vi "Working Lock-In.vi"() -> ()   [LabVIEW 2013, in "Lock-In Variable Channels_2.lvclass"]
uses:
  Lock-In Variable Channels_2.lvclass
  XControl_next Folder/XControl_next.xctl
  Joe's Lock-In Files/Lockin-4461_3.0 4461-4462 Multichannel Folder/DAQ-Lockin-SubVI/Lock-in Globles Multiple Inputs and Outputs.vi
  Joe's Lock-In Files/Global Value_charles.vi
panel:
  out "first_run?":dbl
  out "Phase&Tc Control 2":T1(array[cluster])=[{"Phase"=0.0, "Time constant"=0.1, "Set Tc"=FALSE, "Autophase"=FALSE, "Order"=2.0}, {"Phase"=0.0, "Time constant"=0.1, "Set Tc"=FALSE, "Autophase"=FALSE, "Order"=2.0}, {"Phase"=0.0, "Time constant"=0.1, "Set Tc"=FALSE, "Autophase"=FALSE, "Order"=2.0}, {"Phase"=0.0, "Time constant"=0.1, "Set Tc"=FALSE, "Autophase"=FALSE, "Order"=2.0}, {"Phase"=0.0, "Time constant"=0.1, "Set Tc"=FALSE, "Autophase"=FALSE, "Order"=2.0}, {"Phase"=0.0, "Time constant"=0.1, "Set Tc"=FALSE, "Autophase"=FALSE, "Order"=2.0}, {"Phase"=0.0, "Time constant"=0.1, "Set Tc"=FALSE, "Autophase"=FALSE, "Order"=2.0}, {"Phase"=0.0, "Time constant"=0.1, "Set Tc"=FALSE, "Autophase"=FALSE, "Order"=2.0}, {"Phase"=0.0, "Time constant"=0.1, "Set Tc"=FALSE, "Autophase"=FALSE, "Order"=2.0}, {"Phase"=0.0, "Time constant"=0.1, "Set Tc"=FALSE, "Autophase"=FALSE, "Order"=2.0}, {"Phase"=0.0, "Time constant"=0.1, "Set Tc"=FALSE, "Autophase"=FALSE, "Order"=2.0}, {"Phase"=0.0, "Time constant"=0.1, "Set Tc"=FALSE, "Autophase"=FALSE, "Order"=2.0}, {"Phase"=0.0, "Time constant"=0.1, "Set Tc"=FALSE, "Autophase"=FALSE, "Order"=2.0}, {"Phase"=0.0, "Time constant"=0.1, "Set Tc"=FALSE, "Autophase"=FALSE, "Order"=2.0}, {"Phase"=0.0, "Time constant"=0.1, "Set Tc"=FALSE, "Autophase"=FALSE, "Order"=2.0}, {"Phase"=0.0, "Time constant"=0.1, "Set Tc"=FALSE, "Autophase"=FALSE, "Order"=2.0}, {"Phase"=0.0, "Time constant"=0.1, "Set Tc"=FALSE, "Autophase"=FALSE, "Order"=2.0}] {"Phase" min=0.0 max=360.0 scale=0.0..360.0}
  in  "Boolean_event":bool
  out "Multiple Indicator":bool
  out "Phase indicator":bool
  out "Signal indicator":bool
  out "loop counter":dbl
  out "Amp. button 2":bool
  out "DC button 2":bool
  out "OK Button 2":bool
  out "Boolean_panel3":bool
  out "Boolean_panel2":bool
  out "Numeric_Channel":dbl
  in  "XControl_next":dbl(xcontrol)
  in  "Display":u16(ring) items=["X and Y", "R and Theta"]
  in  "stop":bool
  out "Display 2":string="-000.000000       V"
  out "Display 1":string="-000.000000       V"
  out "Results":dbl[][](array[numeric])=[[1.1085752698169061e-06, 8.970523484593692e-07, 1.426058219262487e-06, 38.9795731407906], [0.009851325382064164, -0.0009794262328395094, 0.009899893308964286, -5.677731707079707], [1.3085970697368273e-06, 7.35860824175527e-07, 1.5013052466038e-06, 29.35026849878307], [2.653910755996262e-06, 1.0145343098285082e-06, 2.8412184299366806e-06, 20.9208047375633], [-6.086289413703597e-07, 1.180787094252328e-06, 1.3284153530528245e-06, 117.2685442231227], [2.777937660299593e-06, 8.877049230863689e-07, 2.9163260577278655e-06, 17.721560078700946]]
  in  "Remote":bool
  out "Backlog":u8(slide) scale=0.0..100.0
  out "Signal":dbl[][](array[numeric])
  in  "Tab Control":T2(tab)=enum."Input Signals"
  in  "Lockin Display A":i16(slide)=1 scale=1.0..18.0
  out "Display X (or R) A":dbl[](graph)=[6.670498573825442e-08, 5.368688471545208e-07, -5.088691339548878e-07, -2.5730186693772355e-06, -1.7991552027288684e-06, -1.923632216975614e-06, -1.4467888340965616e-06, -8.796097429790696e-07, -1.269884182091489e-06, -2.961296758715229e-06, -1.9896471500029525e-06, -2.992785692825242e-06, -1.7650822258067036e-06, -2.6746621457151217e-06, -1.8077634796781362e-07, -2.8403618391177364e-06, 1.7191093719052563e-06, -4.095627199796772e-06, 1.0350053729206764e-07, -3.2952403320842463e-06, 4.027147024255837e-07, -3.217883708836871e-06, -3.1404111038198314e-07, -2.722157981623261e-06, -2.3343431458291097e-06, -1.6493479166701816e-06, -1.1867860941043085e-06, -1.6312467794017544e-06, -1.924154413394931e-06, -1.9805292725153245e-06, 7.32780599223683e-07, -1.9269225043914707e-06, -1.9357725457213794e-06, -2.2334144149538824e-06, -4.935649750003306e-09, -8.436124644364356e-07, -3.307435264761252e-07, -2.3962904127030663e-06, -5.02686543328057e-07, -2.0819204665377523e-07, -6.016691845226929e-07, -3.3346199078653027e-06, -2.3438333439908954e-06, -2.6393322677123663e-06, 4.3707871692753315e-07, -1.955570749471345e-06, -1.0959726290001432e-06, -3.3918492580454637e-06, 2.46039910232935e-07, -1.9940219874551605e-06, -3.6795795043347265e-07, -2.45582698051919e-06, 4.455716118537976e-08, -1.5262074036175926e-06, 2.820130220284548e-07, -1.0569110213571934e-06, -2.3607453703924565e-07, -3.055913228346468e-06, -1.650377972048181e-06, -1.8932005087329695e-06, 5.914078647979998e-07, -1.3508504110029581e-06, -1.7773157019895033e-06, -1.433545330477821e-06, 5.165591171148216e-07, -2.6433445727486453e-07, -5.167671626878888e-07, -6.055573834856804e-07, -3.980981522485872e-07, -9.728044362515663e-07, -1.1758902512983826e-07, -1.6542257074006194e-06, -1.0669038863728946e-06, -1.1680190342438217e-06, -1.4347012124266572e-06, -2.233685467775109e-06, -9.173892627620104e-07, -1.3057567635081897e-06, -5.961972413873471e-07, -1.0467491581646199e-06, -1.5607311611567676e-06, -2.1330252927991802e-06, -1.2651497555792722e-06, -1.5740108560218413e-06, -8.450526108735602e-07, -1.1403712648585578e-07, -1.3527516308023321e-06, -8.078702051960308e-07, -9.409207938670527e-07, -1.5548207904995552e-06, -1.1518398452053984e-06, -1.3918660560555396e-06, -2.0931739723389586e-06, -2.2147164239668027e-06, -3.366260220930173e-06, -1.031323116424528e-06, -6.179742691405814e-07, -2.9460438011649747e-06, -1.1400531118409205e-06, -1.484088446722104e-07, -2.6518751029251362e-06, -4.097924835402338e-07, -2.057919982499709e-06, -2.715956482323881e-07, -6.940554229154257e-07, -7.522735265241387e-07, -7.335964599058371e-07, -2.8600098545973234e-07, -3.4843824827197703e-06, -1.44911890347727e-06, -1.225529253887876e-06, -6.736912990276699e-07, -1.6691842479645122e-06, -2.1938552441526384e-06, -1.4997095470240344e-06, -1.0375533719089362e-06, -1.1301499898056886e-06, -1.4793551793585697e-06, -2.5259160810447276e-06, 3.491557595541023e-07, -1.0993167478065809e-06, -1.068633016308054e-06, -8.806665544284457e-07, 9.238520373506171e-08, -7.19060141525052e-07, -1.22036415098872e-07, -9.144936655123115e-07, -9.321502892559434e-07, -1.8082361748005226e-06, -8.045321826052708e-07, -4.6816599025933015e-07, -1.201527764455396e-06, -9.433090453378502e-07, 5.799679027359041e-07, -2.6489856161776193e-06, 3.022449142514117e-07, 1.1085752698169061e-06, 0.0, 0.0, 0.0, 0.0, 0.0, 0.0, 0.0, 0.0, 0.0, 0.0, 0.0, 0.0, 0.0, 0.0, 0.0, 0.0, 0.0, 0.0, 0.0, 0.0, 0.0, 0.0, 0.0, 0.0, 0.0, 0.0, 0.0, 0.0, 0.0, 0.0, 0.0, 0.0, 0.0, 0.0, 0.0, 0.0, 0.0, 0.0, 0.0, 0.0, 0.0, 0.0, 0.0, 0.0, 0.0, 0.0, 0.0, 0.0, 0.0, 0.0, 0.0, 0.0, 0.0, 0.0, 0.0, 0.0, 0.0, 0.0, 0.0, 0.0, 0.0, 0.0, 0.0]
  out "Display Y (or Theta) A":dbl[](graph)=[1.0286335437287416e-07, 7.146914430049907e-07, 9.19371053154206e-07, -2.7527637468034014e-07, 9.764685600495431e-07, 2.16329849650388e-06, 6.18754045208451e-07, 1.0259603006949609e-06, 2.579095660939101e-07, 1.498736189536387e-06, 1.7791032720161242e-06, 8.722478978782919e-07, 1.179386006030635e-06, 1.3778637608132363e-06, -2.0572071085454253e-07, 7.203248036070591e-07, 6.266561030444089e-07, 1.2536548086139658e-06, -1.6258653973034804e-07, 1.9278115524532664e-06, 5.186481319325723e-07, 8.153605722202512e-07, 5.135548811901674e-07, 1.4550446823081113e-06, 3.3380469223525346e-07, 1.230454826405213e-06, 1.0885651868509204e-06, 1.5786789143860278e-06, 9.455455089747191e-07, 1.2571272379312255e-06, 2.1014333516181865e-06, 6.607774722121163e-07, 4.822838575243949e-07, 9.038988408693548e-07, 1.33469270633984e-06, 6.455872176713377e-07, 5.666811221789705e-07, 1.0640103180436064e-06, 1.4303236294814581e-06, 6.967580372586826e-07, 6.136341751512432e-07, 7.422882569256587e-07, 5.883881949852455e-07, 1.997573203066393e-06, 5.108273813688291e-07, 1.7950225152410556e-06, 1.221042319602369e-06, 9.86349423686866e-07, 9.54101478401993e-07, 1.8534351350083934e-06, 2.2210726847342647e-07, 1.1307278065187195e-06, 1.717119984101465e-06, 1.3768932185795426e-06, 6.851564213751961e-07, 1.5181415571549518e-06, 5.401194326435506e-07, 6.086050050353494e-07, 1.5452845368407302e-06, 6.665165050368888e-07, -8.081778093341734e-07, 6.979796169410442e-07, -1.4355534744700468e-06, 7.933524914480013e-07, -2.0435406862520562e-06, 2.318050967992582e-07, -1.4362641032531598e-06, 1.3131502749455698e-06, -1.4297689132329595e-06, 8.029971520790156e-07, -1.772676282760011e-06, 8.31683435935555e-07, -6.194049516322809e-07, 6.35723502426594e-07, -1.889409421404472e-06, -7.711172640404809e-07, -1.33021114111389e-06, 6.040667275356772e-07, -9.017699433082181e-07, 1.369914851829068e-07, -1.4406998244783337e-06, 4.1440780260440394e-07, -1.0846130485129012e-06, 1.4290306224796054e-06, -2.1346885932959517e-06, 4.736172347707491e-07, -1.188146731611753e-06, 5.466005398577626e-08, -9.135777373074258e-07, 7.456215576100294e-09, -1.5887233604415758e-06, -1.43959584610028e-07, -7.807344692270741e-07, 1.0988391031174632e-06, -1.2935850677734005e-06, 2.6847009001982245e-07, -1.847023978850422e-06, 1.0909219958858604e-06, -1.3075923432183734e-06, 6.612172587787478e-08, -2.137876603499354e-06, -6.15784650222712e-07, 7.731861116125207e-08, 1.0873998539495432e-06, -1.0570344375219628e-06, -1.3484653973993046e-07, -1.269808677468912e-06, -3.2389327137010494e-07, -4.1499635767494345e-07, 9.75014182636857e-07, -1.8805650864728521e-06, 4.329556422464076e-09, -7.299864691271978e-07, 9.51920771580406e-07, -3.2439202609845064e-07, 1.084353022958213e-06, -5.87217042471334e-07, 1.5123484249454393e-06, 6.436642674537832e-07, -6.469642763203526e-07, 2.660240312787005e-07, -1.1561262848561151e-06, 1.6307844515797396e-06, -1.4325815873415714e-06, 9.251531182466132e-07, -1.6623520598966579e-06, 1.978576321169293e-07, -9.142031752824135e-07, 1.3296677206169422e-07, -1.061320726264358e-06, -6.71594978273001e-07, -1.202631936263428e-06, 9.42577383247746e-07, -1.8538521080561355e-06, -3.437941246336895e-07, -8.184972684442104e-07, 8.970523484593692e-07, 0.0, 0.0, 0.0, 0.0, 0.0, 0.0, 0.0, 0.0, 0.0, 0.0, 0.0, 0.0, 0.0, 0.0, 0.0, 0.0, 0.0, 0.0, 0.0, 0.0, 0.0, 0.0, 0.0, 0.0, 0.0, 0.0, 0.0, 0.0, 0.0, 0.0, 0.0, 0.0, 0.0, 0.0, 0.0, 0.0, 0.0, 0.0, 0.0, 0.0, 0.0, 0.0, 0.0, 0.0, 0.0, 0.0, 0.0, 0.0, 0.0, 0.0, 0.0, 0.0, 0.0, 0.0, 0.0, 0.0, 0.0, 0.0, 0.0, 0.0, 0.0, 0.0, 0.0]
  in  "Lockin Display B":i16(slide)=2 scale=1.0..18.0
  out "Display X (or R) B":dbl[](graph)=[0.009851575604636491, 0.009850859603452052, 0.009851399758058718, 0.009851459687556728, 0.00985190891444035, 0.00985226704914683, 0.009850824769245543, 0.009852235734838408, 0.009851610294980736, 0.009850813605968936, 0.009851284837196808, 0.009851241662153556, 0.009851271919100256, 0.009850614652581096, 0.009851407933718264, 0.009852094491344282, 0.009850578046171154, 0.009851695944019327, 0.009850881878743124, 0.009851234272305626, 0.009851365691234364, 0.009850433177655573, 0.009850796883405188, 0.009851143432907442, 0.009850939980893697, 0.009851121609399043, 0.009850912546900518, 0.009851247859729465, 0.009851202852210975, 0.009851545715095328, 0.009851306348303227, 0.009851317442401263, 0.009850760256779275, 0.009851745232648836, 0.00985186673671429, 0.009850025057442865, 0.009851213088299709, 0.009851396764747646, 0.009850759672557035, 0.009850957869685937, 0.00985145652409099, 0.009850986942748257, 0.009850401960925475, 0.009850992493070105, 0.009850894547177688, 0.009850505369384019, 0.009851878887673884, 0.009850544792531387, 0.009851942371396335, 0.009850555088563345, 0.009852138529925395, 0.009852231920765613, 0.009851180635846068, 0.009851195406466975, 0.00985063841729186, 0.009850913455266373, 0.009851042413661481, 0.009850265865374463, 0.009851555351183676, 0.0098513031551279, 0.009851193362171287, 0.009851189052643577, 0.009849897577948696, 0.009851468711997591, 0.009851836020381127, 0.009850864598215292, 0.009850036913672594, 0.009851237936284942, 0.009851381092893002, 0.009850999119045252, 0.009850910401055669, 0.00985116377967753, 0.009850712333951097, 0.009850492008067039, 0.009851138183793956, 0.0098520738676251, 0.009850647490696045, 0.009850219592452195, 0.009850698028558178, 0.009851360930690974, 0.009851308016245243, 0.009850591670241656, 0.009850782078694142, 0.009851107550509084, 0.009850499265131867, 0.009851601588433817, 0.00985200817802394, 0.00985161281126096, 0.009851229915089514, 0.009851057719900627, 0.009850538907064495, 0.009850398907869583, 0.009851390570047658, 0.009851944298770189, 0.009850861750384889, 0.009851845513163027, 0.009850996943534297, 0.009851407105435486, 0.009851443172057484, 0.00985013354071063, 0.009851331696312308, 0.00985155962884771, 0.009851937178113734, 0.009850569661817103, 0.00985141722120437, 0.009851856785726667, 0.009850984175157314, 0.009849882615623187, 0.00985117161929196, 0.009850528217824051, 0.009851269147894678, 0.009850740429011275, 0.009851115241466393, 0.009851657412155707, 0.009850618670449616, 0.009850849040852393, 0.00985058695171117, 0.00985129559098424, 0.009851414197706507, 0.009850223948569119, 0.009852184547009205, 0.009851653747128136, 0.009850889570269934, 0.009850965207748103, 0.00984986780199983, 0.009851378038917103, 0.009851254489611947, 0.009850175106914542, 0.00985146363681588, 0.009851464694800242, 0.009850663048481277, 0.009850868296036626, 0.009851106055751357, 0.009851402847979952, 0.009851127890145413, 0.009851839949532912, 0.009851325382064164, 0.0, 0.0, 0.0, 0.0, 0.0, 0.0, 0.0, 0.0, 0.0, 0.0, 0.0, 0.0, 0.0, 0.0, 0.0, 0.0, 0.0, 0.0, 0.0, 0.0, 0.0, 0.0, 0.0, 0.0, 0.0, 0.0, 0.0, 0.0, 0.0, 0.0, 0.0, 0.0, 0.0, 0.0, 0.0, 0.0, 0.0, 0.0, 0.0, 0.0, 0.0, 0.0, 0.0, 0.0, 0.0, 0.0, 0.0, 0.0, 0.0, 0.0, 0.0, 0.0, 0.0, 0.0, 0.0, 0.0, 0.0, 0.0, 0.0, 0.0, 0.0, 0.0, 0.0]
  out "Display Y (or Theta) B":dbl[](graph)=[-0.000963633864588737, -0.000979286079411311, -0.0009796988273423545, -0.000979639218807666, -0.0009790557079538752, -0.0009799921233401507, -0.0009803696532139565, -0.0009802652128818303, -0.000979965328011669, -0.0009796685184549605, -0.0009797371501994293, -0.0009799903281541235, -0.0009800009104722533, -0.0009796771131844236, -0.0009791973852113724, -0.0009793284320958283, -0.0009802697916852774, -0.0009798876216329348, -0.0009790558850193212, -0.0009799295750890346, -0.0009808315171088568, -0.0009800027763974231, -0.0009798662309455056, -0.0009794699138142556, -0.0009800191817064922, -0.0009787592796008657, -0.000980079551444322, -0.0009799888125970712, -0.0009795353655923716, -0.0009794323127544319, -0.00097950280529945, -0.0009801793902978195, -0.000979494306836292, -0.0009803223619375483, -0.000979637794480237, -0.000979885100980701, -0.0009798880685902742, -0.0009796998883248242, -0.0009793919209932851, -0.0009795581867642574, -0.0009795490839255207, -0.0009795982076275665, -0.000980278704664193, -0.0009797372836355884, -0.0009792479263135375, -0.0009792502055057514, -0.0009790689943955915, -0.0009800576636865386, -0.0009795733062281339, -0.000979280339659147, -0.0009788067331125223, -0.000979911583012091, -0.0009798824626715168, -0.0009795471950167893, -0.0009790609377079071, -0.0009797287572532853, -0.0009794720232180715, -0.0009796045750319366, -0.0009797411272829408, -0.0009804487893015513, -0.00098004263004027, -0.000980734680871649, -0.000979727442777383, -0.000979461546970301, -0.0009795791465842245, -0.0009804982536090715, -0.0009799347993178719, -0.0009794563261029555, -0.0009789411958013234, -0.0009793112210103334, -0.0009799646236544677, -0.0009797525907774764, -0.0009793973052425035, -0.000979764586325322, -0.000980066005499762, -0.0009798744199403418, -0.0009793435327893716, -0.0009785579838452808, -0.000980230697116573, -0.0009803011619646152, -0.0009801748027126918, -0.0009800867104999811, -0.000979817063271664, -0.000979541092234591, -0.0009795855509299634, -0.0009799872559213166, -0.0009791072009137653, -0.0009800249080251257, -0.0009794881841494148, -0.0009802606987228766, -0.0009802483846104095, -0.0009803318816857475, -0.0009800448616099433, -0.0009795793172353545, -0.000979643918858572, -0.0009793660029603249, -0.0009796891336956539, -0.0009796736571797155, -0.0009801053201216484, -0.0009797060769168651, -0.0009798437933049508, -0.000979133925260368, -0.000979992798406434, -0.0009806152554006791, -0.0009787731648931617, -0.0009796545242979555, -0.0009796277365916597, -0.0009791825568666748, -0.0009792062550888314, -0.000980059673274802, -0.0009806751636411818, -0.000979253881350918, -0.000978913926006237, -0.000979578792464132, -0.0009800177517536814, -0.0009796951825853154, -0.000979354022084312, -0.000979444922776568, -0.0009799988953658957, -0.0009789005180601623, -0.0009802443305960264, -0.0009801161941698092, -0.0009796448924835567, -0.000979179862632047, -0.0009791942851141563, -0.0009796150304151453, -0.0009798424293192742, -0.0009790224229659246, -0.0009794452768922353, -0.0009800891849019648, -0.0009795693582131944, -0.000979663422779722, -0.0009795835163406807, -0.0009790433466292203, -0.0009797819678512916, -0.0009798142535752152, -0.0009794262328395094, 0.0, 0.0, 0.0, 0.0, 0.0, 0.0, 0.0, 0.0, 0.0, 0.0, 0.0, 0.0, 0.0, 0.0, 0.0, 0.0, 0.0, 0.0, 0.0, 0.0, 0.0, 0.0, 0.0, 0.0, 0.0, 0.0, 0.0, 0.0, 0.0, 0.0, 0.0, 0.0, 0.0, 0.0, 0.0, 0.0, 0.0, 0.0, 0.0, 0.0, 0.0, 0.0, 0.0, 0.0, 0.0, 0.0, 0.0, 0.0, 0.0, 0.0, 0.0, 0.0, 0.0, 0.0, 0.0, 0.0, 0.0, 0.0, 0.0, 0.0, 0.0, 0.0, 0.0]
  in  "Lockin Display C":i16(slide)=3 scale=1.0..18.0
  out "Display X (or R) C":dbl[](graph)=[-9.745747368487622e-07, 2.353099020423567e-07, -5.42338939801975e-07, -4.718986842457581e-07, -7.593538186286168e-07, -1.7952022845519822e-06, 1.0142878386372215e-06, -9.274394581256076e-07, 1.7372756519437092e-07, -6.985181798404725e-07, -4.731782746944689e-07, -8.846505321399338e-07, 1.13049206100105e-06, -2.390760772040696e-06, -2.840973100331342e-07, -8.38467648834523e-07, 1.108902128041089e-06, -1.6039202249658034e-06, 1.0588651240934854e-06, -5.121521295546275e-07, 8.893208384019807e-07, -1.6492728245965068e-06, 1.6712442373602972e-08, -8.566336995531172e-07, 7.77824876530707e-07, -1.2325010132965547e-06, -1.222430436285416e-06, -1.128224113439429e-06, 1.5380793762595435e-06, -4.818705059571917e-07, 1.8576468066427286e-07, -6.96848132866836e-07, 4.458332977509825e-07, -6.810902878584071e-07, 1.963579866623903e-06, -1.1181604976967486e-07, 9.70993024601419e-08, -1.2240598315532683e-06, 1.0086955767278806e-06, -6.920279328337381e-07, 7.03649456116012e-07, -1.5504344163842393e-06, -1.1295936237214322e-06, -1.4693816328148374e-06, 1.2396993755364977e-06, -4.3991070221885074e-07, -1.6824942607002498e-07, -3.6156093603475506e-07, 1.2834901648389448e-06, -2.284542107972361e-06, 4.4476291419760956e-07, -1.3280505347429105e-06, 1.0303097816146845e-06, -5.512245340294317e-07, 1.6165308841022732e-06, -1.6303654168061304e-06, 6.464116355230595e-07, -5.036585833189266e-07, 3.2179642771582177e-07, -1.29269475045368e-06, 8.936789963890076e-07, -3.699661980073172e-07, 1.6526513695269567e-06, 7.596670069936549e-08, 4.023708834018227e-07, -4.840055224201998e-07, 9.605812613473206e-07, -1.385304993402932e-06, 6.924517928224892e-07, 3.964460847682789e-07, 6.798901732029211e-07, -5.702247225593159e-07, -9.776670041562167e-07, -1.4535685877954301e-07, -1.8165762178952627e-07, 6.520930313105914e-08, 5.315046326034288e-07, -5.390711813688558e-08, 5.772657010873898e-07, -7.869913508628625e-07, -1.1007054933886128e-06, -1.3179443571970436e-06, -9.886921119301582e-07, 2.473538031061813e-07, -2.8309193408455994e-07, 5.71585834230155e-07, -1.2738806140609586e-06, 3.3975677278817674e-09, 1.546000653443958e-07, -1.305925732832836e-07, -1.3450144320517078e-06, 2.610439814225301e-08, -4.949145579678015e-07, 9.286062035234121e-07, -1.3380391194425453e-06, 2.3628037423973685e-07, 5.862037191205384e-07, -1.4197807617625318e-06, -1.618688068932426e-06, -3.817861805373953e-08, -1.0117870528168358e-06, 1.140620456765397e-06, -6.577971292048741e-07, 6.638683303164139e-07, -6.874759327955524e-07, -3.0571223131595493e-07, -1.4634373232658826e-06, 4.6369946461187475e-07, -1.3476568182938803e-06, -2.7956018300582267e-09, -3.438798197982888e-08, -5.181968854795809e-07, -6.867910171256003e-07, 9.124957549964032e-08, -1.0785242713378164e-06, 7.101402235370799e-08, -8.566659645075696e-07, 3.764105431329948e-07, -2.1463308938479247e-06, 3.0267109176652875e-06, -4.301805387335276e-07, -5.218305950810351e-07, 2.153441987414774e-06, 1.3547626370499898e-06, 5.113445364631065e-07, -3.365971693824349e-07, -2.4092387942846915e-08, 5.50304606088644e-07, 3.3424418305986044e-07, 6.77152848593253e-07, -3.080043884239647e-08, 1.1790378979431875e-06, -7.015863231814383e-07, 6.714311549584288e-07, -1.080633929845727e-06, 1.4107562551154975e-06, 1.3085970697368273e-06, 0.0, 0.0, 0.0, 0.0, 0.0, 0.0, 0.0, 0.0, 0.0, 0.0, 0.0, 0.0, 0.0, 0.0, 0.0, 0.0, 0.0, 0.0, 0.0, 0.0, 0.0, 0.0, 0.0, 0.0, 0.0, 0.0, 0.0, 0.0, 0.0, 0.0, 0.0, 0.0, 0.0, 0.0, 0.0, 0.0, 0.0, 0.0, 0.0, 0.0, 0.0, 0.0, 0.0, 0.0, 0.0, 0.0, 0.0, 0.0, 0.0, 0.0, 0.0, 0.0, 0.0, 0.0, 0.0, 0.0, 0.0, 0.0, 0.0, 0.0, 0.0, 0.0, 0.0]
  out "Display Y (or Theta) C":dbl[](graph)=[-7.463915153616716e-07, 8.189966377917778e-07, 1.023125302989645e-06, -3.9007387655037716e-07, 1.0520302133887266e-06, 1.5758254298913815e-06, 5.161875423223932e-07, 1.1727418576025086e-06, 1.2982846579056094e-06, 1.3797862385654182e-06, 1.7214845208450932e-06, 1.7936224874337971e-06, 8.941765712750468e-07, 2.252742789385369e-06, 6.011344214109727e-07, 9.842809102578028e-07, 4.427116837872148e-07, 1.4040169378778715e-06, -8.602147514592055e-07, 1.6464364696866766e-06, 1.071305825942507e-06, 7.008837258931724e-07, 9.508746458565877e-07, 1.7202730618749724e-06, 6.092432033706318e-07, 1.3331707768507746e-06, 1.8708901901382738e-06, 8.310793132238205e-07, 8.610097241214849e-07, -3.501561363499112e-07, 4.800840215051806e-07, 8.522113464513712e-07, 1.6829950348137602e-06, 1.6141441124754706e-06, 1.4462169807749354e-06, 1.0364807194285358e-06, 4.425637875412655e-07, 1.5841692429554045e-06, 1.046673896532509e-06, 1.0925483212375711e-06, 2.844804874492595e-07, 1.092982115223684e-06, 3.7882000670584364e-07, 5.211905535721634e-07, 9.859656315643583e-07, 1.7965868266825963e-06, 4.543234760667269e-07, 1.4115620698856758e-06, 8.310615169213983e-07, 6.897422760679255e-07, 1.3446151038886205e-07, 1.0550110488986515e-06, 1.2988007238403532e-06, 1.5251747619802425e-06, 3.3689605455235815e-08, 1.213874933020901e-06, 1.2489586121249465e-06, 6.037584522671578e-07, 1.684062323353709e-06, 8.854034875865685e-07, -3.0286991289630804e-07, 7.469348340186213e-07, -8.860449233568259e-07, 9.346225122903532e-07, -1.5044905423379502e-06, -2.6327870533692464e-07, -8.764513772078728e-07, 2.924372673419274e-07, -1.1728500569618128e-06, -6.540453726365163e-07, -1.1699238702348134e-06, -3.4781532310340924e-08, -2.3971884623143614e-06, 6.349203578371252e-09, -1.439538509531894e-06, -2.454067687407202e-07, -5.739833285624475e-07, 3.408314241252573e-07, -9.75835623064447e-07, 4.3749439407959864e-07, -1.148649034166207e-06, 9.96581688311274e-07, -1.1465283383125819e-06, 9.455204476734759e-07, -1.8077216932368424e-06, 7.278213996541632e-07, -1.6400300368749656e-06, 4.2808424871860765e-08, -1.4328812270379611e-06, 6.494938923458857e-07, -2.249141038709575e-06, 4.25028670530157e-07, -5.495642692738775e-07, -1.4835927540573295e-08, -1.4091168703570004e-06, 4.824385194713739e-07, -1.8864769116883122e-06, 1.017426909062845e-06, -5.766249278237553e-07, -2.7237433520927516e-07, -1.7527468606995399e-06, -2.492667712876311e-07, -1.3656852780302997e-06, 1.5259936161919402e-06, -1.394675779400796e-06, -2.5004485399218825e-07, -7.761456844127054e-07, 6.689297001779621e-07, -2.749065137561659e-07, 4.1293822715596605e-07, -4.927915833475579e-07, 7.514162636747805e-08, -6.094966535434958e-07, 1.0208834265104418e-07, -7.634004209235431e-07, 5.07812517258729e-07, -1.116386366278656e-06, 5.657615694708508e-07, 6.568049442627294e-07, 1.2125257392448532e-07, 1.1075396280592844e-06, -3.3358516087632676e-07, 9.488473251926233e-07, -1.1459501771008652e-06, 5.8730064061527366e-08, -1.6415932922799296e-07, 4.851760627048216e-07, -2.7152481986597594e-07, 1.5770472588038617e-07, -1.3777935285459273e-06, 1.8112303061219635e-07, -1.230007897568607e-06, 1.1870334606424432e-06, 4.437877774782821e-08, 1.8141072069395773e-07, -6.297945866741428e-09, 7.35860824175527e-07, 0.0, 0.0, 0.0, 0.0, 0.0, 0.0, 0.0, 0.0, 0.0, 0.0, 0.0, 0.0, 0.0, 0.0, 0.0, 0.0, 0.0, 0.0, 0.0, 0.0, 0.0, 0.0, 0.0, 0.0, 0.0, 0.0, 0.0, 0.0, 0.0, 0.0, 0.0, 0.0, 0.0, 0.0, 0.0, 0.0, 0.0, 0.0, 0.0, 0.0, 0.0, 0.0, 0.0, 0.0, 0.0, 0.0, 0.0, 0.0, 0.0, 0.0, 0.0, 0.0, 0.0, 0.0, 0.0, 0.0, 0.0, 0.0, 0.0, 0.0, 0.0, 0.0, 0.0]
  in  "Lockin Display D":i16(slide)=4 scale=1.0..18.0
  out "Display X (or R) D":dbl[](graph)=[1.2164728075488221e-06, 5.588663742450228e-07, 6.872801892487782e-07, -1.2985657907644942e-06, -8.614491119275728e-08, -1.9002255709597074e-06, -1.110924600299573e-06, -1.4695526420666973e-06, 8.442181959601978e-07, -2.7261280075085316e-06, -1.1319639442024771e-07, -1.0429663332276367e-07, -6.045137345984591e-07, -2.4877023314287054e-06, 5.240644398570024e-07, -1.7822075361445778e-06, 1.5413748183912478e-06, -1.2897976737523536e-06, 1.8854766221200609e-06, -1.6266072945853216e-06, 1.7616195593293483e-06, -2.2275000449394434e-06, 5.687459713123476e-07, -5.389750317030624e-07, 4.0405997349394546e-08, -1.54737867663715e-06, -9.527376377132272e-07, -9.914360194064139e-07, -3.851381910682226e-08, -5.509617449399491e-07, -1.9332554847273088e-07, -1.9830623713016993e-06, 4.998902080355647e-07, -2.8638150477873875e-07, 2.630681196278918e-07, -1.2526174640047816e-07, 6.870894858900778e-07, -1.8334354877372318e-06, 2.196417127225883e-06, -9.73210337059156e-07, 8.746703866726511e-07, -5.128144124883403e-07, -9.315527946656625e-07, -1.6973333804140617e-06, 1.1063706585655493e-06, -1.4314942206751845e-07, 3.7572082964579033e-07, -7.523404184235564e-07, 5.812545519203096e-07, 3.716781921557211e-08, 1.655176055412939e-06, -1.3341908932203386e-06, 2.4307977747041766e-07, -7.750986698414027e-07, 1.0707296519645986e-06, -1.835125786073871e-06, 1.3641445131525142e-06, -6.324851423318175e-07, 7.560576475020995e-08, -8.590224006587895e-07, 1.8945582092189254e-06, -9.7355814332125e-07, 1.8348694181962466e-08, -8.670985835386837e-07, -5.178043949145894e-07, 1.0617953172762162e-06, 9.225519298987308e-07, -7.012712592591851e-07, 3.5792512274961327e-07, 1.2561571378945572e-06, 8.838459346563438e-08, -1.6801943289520777e-06, -6.566571034865103e-07, 3.235319894209203e-08, -8.637870319170892e-07, -6.985095474015429e-07, 1.17965563354636e-07, 7.234528778971199e-07, 6.218867435886975e-07, 6.710271822873673e-07, 1.1051208706824134e-07, -5.34409276130322e-07, -7.698024164378941e-07, -1.0508972056087116e-06, -5.393053173829247e-07, 5.24360875443029e-07, 1.1438986132671824e-07, -5.61565428377689e-07, 3.731932473906685e-07, -4.052339212247889e-07, 7.881701115277939e-07, -1.0642139668652509e-06, -2.97443954005839e-07, -1.0293012524082224e-06, -8.519297431507719e-07, 2.2139875315257238e-07, -5.925500625300188e-07, -1.6179864859883432e-06, 5.45548591097003e-07, -7.512449193302707e-07, -7.403527576597557e-07, -7.34474551511069e-07, 5.1824450792798704e-08, 2.373478099816125e-07, -1.6241709509225598e-06, 1.8041367274123543e-08, -5.432169581657867e-07, -1.122359060074928e-06, -6.804956625137456e-07, -2.1883488438339897e-07, -1.0285640857202739e-06, -1.435864564712281e-06, 5.848937458792489e-07, -1.0808245957972273e-06, -8.6937837871134e-07, -5.514796543606162e-07, -3.565353281309956e-07, -5.337918405342055e-07, -1.0402065350927625e-06, 1.9020874422060308e-06, 2.661053121974946e-07, 5.432879596854366e-07, 8.992600306888615e-07, 1.8522379837987619e-06, -8.573666108146585e-07, 6.75390090570743e-07, -6.539999675627107e-07, -5.361405384351719e-07, -6.666471052379888e-07, 5.956185074226499e-07, -4.86566783595473e-07, 1.3524676854098565e-06, -8.129172147442943e-07, 1.392569512488896e-06, -1.5871348100276985e-07, 1.4029364775018139e-06, 2.653910755996262e-06, 0.0, 0.0, 0.0, 0.0, 0.0, 0.0, 0.0, 0.0, 0.0, 0.0, 0.0, 0.0, 0.0, 0.0, 0.0, 0.0, 0.0, 0.0, 0.0, 0.0, 0.0, 0.0, 0.0, 0.0, 0.0, 0.0, 0.0, 0.0, 0.0, 0.0, 0.0, 0.0, 0.0, 0.0, 0.0, 0.0, 0.0, 0.0, 0.0, 0.0, 0.0, 0.0, 0.0, 0.0, 0.0, 0.0, 0.0, 0.0, 0.0, 0.0, 0.0, 0.0, 0.0, 0.0, 0.0, 0.0, 0.0, 0.0, 0.0, 0.0, 0.0, 0.0, 0.0]
  out "Display Y (or Theta) D":dbl[](graph)=[-2.5195087038166464e-07, 8.921703037770725e-07, 9.867102928247133e-07, 5.166532713148387e-07, 1.6069757770980633e-06, 8.995365717826155e-07, 8.77326417908995e-07, 6.539515817901696e-07, 1.291414032693513e-06, 1.1900985607130685e-06, 1.0750827693025682e-06, 2.8825878917558555e-08, -1.4578194364816388e-07, 1.2589224585944863e-06, 5.71759438283503e-07, 1.292650551182615e-06, 8.952622113493717e-07, 5.203478657512992e-07, -6.766931287480149e-07, 1.075269826836709e-06, -3.142171073121339e-07, 1.1559515585039385e-07, 1.0309389566437296e-06, 1.6875367694454555e-06, 5.137103507160235e-07, 2.357707288393624e-06, 3.0767495809962795e-07, 6.022570304622383e-07, 1.6280839227388363e-07, 9.464504561202383e-07, 1.5934727763984213e-07, 4.894652981384948e-07, 1.1289088841534937e-06, 2.444036170794044e-06, 1.0777623908849299e-06, 4.6926513143840195e-07, 8.628380497031084e-07, 8.142371913500096e-07, 8.144480799652294e-07, 1.5745739464297088e-07, 1.2554142821113584e-08, 8.639056950664253e-07, 1.2622244471787252e-07, 1.1003971366884816e-06, 1.889971245193138e-07, 1.6931805867206876e-06, 6.359982875555696e-07, 2.2990987951435844e-07, 1.1225019457626219e-06, 7.69905065120756e-07, 4.596159649180705e-07, 9.203487470379476e-07, 6.298491894317466e-07, 8.932180562500768e-07, 6.983677282500886e-07, 1.09209806391265e-06, 2.9615038327784616e-07, 7.742702482119985e-07, 1.164459096154505e-06, 1.550975488162971e-06, -4.3730919659627914e-08, 4.1114815908452263e-07, -4.3183323122914903e-07, 7.427248026646676e-08, -8.062640914024879e-07, 4.168270268913843e-07, -2.0838024646103515e-06, -3.440950183744515e-07, -9.136152964592069e-07, -3.048950121658327e-07, -2.4780373941169076e-06, -7.694910780213594e-08, -4.502349718417997e-07, 8.5709295796942e-07, -2.393380273603818e-06, 4.0277046053961385e-07, -1.225540191441525e-06, 1.4686938811838614e-07, -1.750245526203442e-06, 4.195840560393582e-07, -2.3484664414474707e-06, 9.898895803493653e-08, -9.552756984696104e-07, 5.442211116819632e-07, -1.1866980490560634e-06, 3.315010711927591e-07, -1.4643343031134765e-06, 1.8898574643022458e-07, -3.464751939694818e-07, -2.462243090695094e-07, -1.8700504825980667e-06, 3.3672357606205105e-07, -1.3291532240574156e-06, 6.706948339607724e-07, -5.263414428133967e-07, 1.0894369737881073e-06, -2.087698747915761e-06, 7.169714607335142e-07, -9.779661254693935e-07, 6.153928086894803e-07, -1.4179264284883034e-06, 8.700322205618643e-08, -8.647076247739422e-07, 7.891432067935643e-07, -3.74524471414228e-07, -4.963327394552725e-07, -1.5525895473710555e-06, 7.491225041476924e-07, -5.611966381197367e-07, -2.552442406024144e-07, -1.3227923359753187e-06, -6.926005021778078e-08, 4.6773326506324346e-07, 1.186230185481105e-06, 7.353603110988713e-07, 1.3311868915943158e-06, -2.7041465490739572e-08, 8.108531671943304e-07, 7.491642386145434e-07, 1.1832857656648501e-08, 7.303834886988927e-07, 4.798650572296925e-07, 1.347043846514807e-06, -1.5536670681203177e-06, 7.937955226583783e-08, -7.039114026792199e-07, 2.771748089850597e-07, -1.4727935027226591e-06, -9.270050878135177e-07, -8.24529781161334e-07, 2.7381539426259183e-07, -1.7235553869716161e-07, 1.5022329459353535e-06, -2.6822424397664025e-07, -8.841794009997392e-09, -1.1641264286086446e-06, 1.0145343098285082e-06, 0.0, 0.0, 0.0, 0.0, 0.0, 0.0, 0.0, 0.0, 0.0, 0.0, 0.0, 0.0, 0.0, 0.0, 0.0, 0.0, 0.0, 0.0, 0.0, 0.0, 0.0, 0.0, 0.0, 0.0, 0.0, 0.0, 0.0, 0.0, 0.0, 0.0, 0.0, 0.0, 0.0, 0.0, 0.0, 0.0, 0.0, 0.0, 0.0, 0.0, 0.0, 0.0, 0.0, 0.0, 0.0, 0.0, 0.0, 0.0, 0.0, 0.0, 0.0, 0.0, 0.0, 0.0, 0.0, 0.0, 0.0, 0.0, 0.0, 0.0, 0.0, 0.0, 0.0]
  out "Input Signal":dbl[][](graph)
  in  "Input Signals":i16(slide)=1 scale=1.0..20.0
  out "Phase Log":dbl[](array[numeric])=[0.9999999999893834, 0.9999999999893834]
  out "Sampling Information":cluster{"Fs":dbl, "#s":dbl}[](array[cluster])=[{"Fs"=10000.0, "#s"=5000.0}, {"Fs"=10000.0, "#s"=5000.0}]
  out "AO Task":refnum<k21>[](array[refnum])
  out "AI Task":refnum<k21>[](array[refnum])
  in  "Tab Control 2":T3(tab)=enum."Lock-In Settings"
  in  "Max AI Rate Control":i32=10000
  in  "Auto Control Max AI Rate/AI Block Size":bool=TRUE
  in  "AI Buffer Size (s) Control":i32=100
  in  "AI Block Size Control":i32=5000
  out "AI Rate":dbl=10000.0 format="%.2f"
  in  "AI Configuration Control":T4(array[cluster])=[{"AI.Coupling"=10050, "AI.Max"=10.0, "AI.Min"=-10.0, "Input physical channels"="Dev2/ai0"}] {"AI.Coupling" items=["AC"=10045, "DC"=10050, "GND"=10066]}
  in  "AO Configuration Control":T5(array[cluster])=[{"Output physical channels"="Dev2/ao0", "AO. Max"=0.1, "AO.Min"=-0.1}]
  in  "Numeric_OSC":dbl
  in  "Next_OSC":bool
  in  "Previous_OSC":bool
  out "Numeric_Card":dbl
  in  "Next_Card":bool
  in  "OSC Configuration Control":T6(array[cluster])=[[{"Signal Type"=enum."Triangle Wave", "DC"=0.0, "Amplitude"=0.00799999999999999, "Frequency"=20.0, "Phase"=0.0}]] {"Frequency" step=0.001 format="%.3p"; "Amplitude" format="%0.2p"; "DC" min=-0.99 max=0.99 format="%.2p"}
  in  "Phase&Tc Control":T7(array[cluster])=[{"Phase"=91.58426145861418, "Time Constant"=0.0, "Set Tc"=FALSE, "Autophase"=FALSE, "Order"=0.0}] {"Phase" min=0.0 max=360.0 scale=0.0..360.0}
  in  "Previous_Card":bool
  in  "Next_Channel":bool
  in  "Previous_Channel":bool
  in  "freq. button":bool
  in  "DC Button":bool
  in  "Amp. button":bool
  in  "Signal Button":bool
  in  "Phase Button":bool
  in  "Multiple Button":bool
  in  "Mode Selection":enum32{"Continuous", "Trigger Mode"}(radio)
  in  "Trigger Parameter":u16(ring) items=["DC", "Frequency", "Amplitude", "Signal Type", "Phase", "Multiple Parameter"]
  in  "Data Control":u16(ring) items=["Interactive", "Programmatic"]
  in  "Read initial settings from:":bool
  # "need to check that this works for\ntwo usb-4431s at the same time"
  # "usb - 4431 \nrunning in cont. deletes the\nphase array, you need to initialize again"
  # "this doesn't happen outside of the USB-4431"
  # "something in the get reference for demodulation\nis destroying the phase and time constant array\nwhen the program first starts, but it doesn't \nhave the same effect when you start the\nprogram first and then change the Phase&Tc\narray"
  # "solved using a loop counter and another variable\n-need to check that this works for non-USB 4431\nthings"
  # "-clean up wires/comment"
  # "-email to myself both latest lock-in and van der pauw\n-email to patrick with both attached and the locations on disk\nof the lock-in program as well"
  # "Configurations"
  # "Lock-In Configurations"
  # "Trigger:"
  # "Card (rows)"
  # "Channel (columns)"
  # "note: there must \nbe a Phase&Tc\narray corresponding\nto each channel you\nare using"
  # "Trigger Configurations"
  # "Trigger Settings:"
  # "note: single parameter changes\ncan be made in multiple\ncards/channels as long as\nit is the same parameter\nin interactive mode"
  # "note: for interactive lock-in must run locally\n           for programmatic lock-in must run remotely"
  # "Programmatic Settings:"
  # "Additional Notes:\n-when triggering interactively from the user interface, enter\nthe value change, press enter, and then press the correct button\nto trigger the lock-in; if you don't press enter, the\nlock-in has a tendency to miss the trigger for some reason \nand will not update\n-you will get an odd looking graph when you run the program for the\nfirst time after loading and none of the data will be send to the\nglobal variable; you need to run a second time, i.e. stop and restart the\nprogram and it will self-correct\n-using the USB-4431, if you get a odd-looking graph or the program \nproduces an error, you may need to increase the AI buffer size\n-the interactive trigger mode does not work for the USB-4431"
  # "Instructions and Update History"
  # "Features:\n1, Any number of input and output channels\n2, Each AO outputs an DC+AC signal, DC for sample biasing and AC for OSC. These values can be adjusted in real time.\n3, Synchronous filtering\n\nInstructions:\n1, Array index of AI configuration and AO configuration refers to task.\n2, Array index in Amplifier Settings, Phase$&Tc control , and gains correlates to channel number.\n3, Each 4461 board can have 2 lock-in channels. Syntax for 2 channles, e.g. PXI1Slot2/ai0:1. If you want to use just one, then PXI1Slot2/ai0.\n4, Parameters (especially DC value for sample biasing) can be remotely controlled by clicking \"local\"and \"remote\" button. In real experiments, put golable values (can be found in Lock-in globles.vi) in your VI to control the lock-in and read out.\n5, choose OSC frequencies to be multiple of \nAI Rate/AI Block SIze to have best performance.\n-Guanglei 06/23/2011\n\nUpdate:\n1. Allows any number of lockin amplifiers and AO tasks.\n2. Delete the channels from any AI/AO Configuration elements you do not want to use.\n3. Rows (first index) of the OSC Configuration correspond to different AO tasks, while columns (second index) correspond to AO channels in that task. All channels in a given element of the AO Configuration array will go into a single task.\n4. The same number of output channels must go in each AO task.\n5. Make sure a Phase&Tc element and an Amplifier Settings element is set for each AI channel.\n-Joe 12/3/2013\n\nUpdate (v.2)\n\n1. Works with up to 8 cards/USB devices (can add more but need to hardwire more cases into the program in the Read and Return AO Task.vi)\n2. Dynamic start button, next/previous navigation buttons (only in continuous mode) added\n3. Trigger Mode-interactive and programmatic-added (interactive mode doesn't work with the USB-4431)\n-Charles Law 8/1/2014"
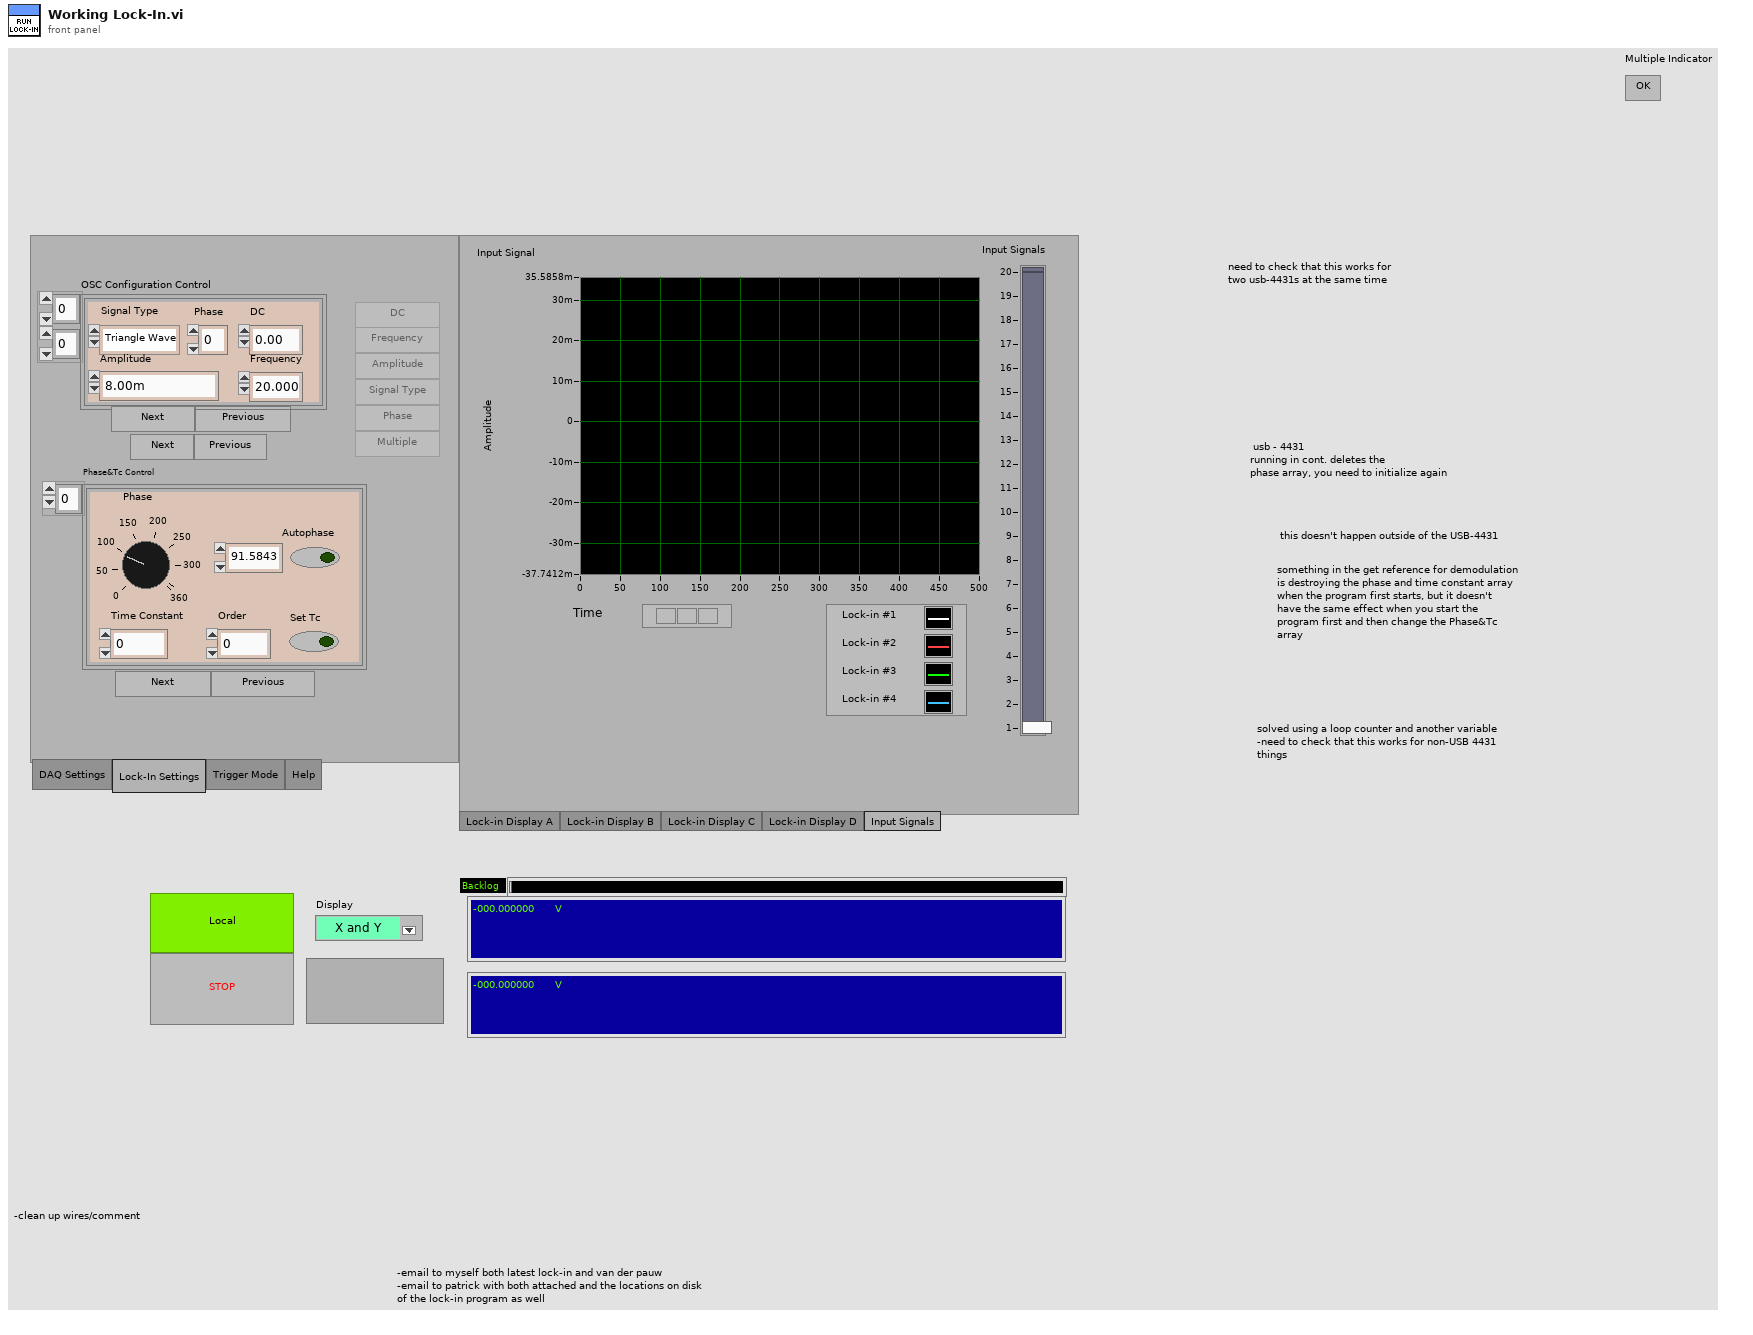
[diagram p1: front panel]
types:
  T1 = cluster{"Phase":dbl, "Time constant":dbl, "Set Tc":bool, "Autophase":bool, "Order":dbl}[]
  T2 = enum32{"Lock-in Display A", "Lock-in Display B", "Lock-in Display C", "Lock-in Display D", "Input Signals"}
  T3 = enum32{"DAQ Settings", "Lock-In Settings", "Trigger Mode", "Help"}
  T4 = cluster{"AI.Coupling":i32, "AI.Max":dbl, "AI.Min":dbl, "Input physical channels":tag}[]
  T5 = cluster{"Output physical channels":tag, "AO. Max":dbl, "AO.Min":dbl}[]
  T6 = cluster{"Signal Type":enum16{"Sine Wave", "Triangle Wave", "Square Wave", "Sawtooth Wave"}, "DC":dbl, "Amplitude":dbl, "Frequency":dbl, "Phase":dbl}[][]
  T7 = cluster{"Phase":dbl, "Time Constant":dbl, "Set Tc":bool, "Autophase":bool, "Order":dbl}[]
  T8 = enum8{"Enabled", "Disabled", "Disabled and Grayed Out"}
  T9 = cluster{"Signal Type":enum16{"Sine Wave", "Triangle Wave", "Square Wave", "Sawtooth Wave"}, "DC":dbl, "Amplitude":dbl, "frequency":dbl, "Phase":dbl}[][]
  T10 = cluster{"Signal Type":enum16{"Sine Wave", "Triangle Wave", "Square Wave", "Sawtooth Wave"}, "DC":dbl, "Amplitude":dbl, "Frequency":dbl, "Phase":dbl}
  T11 = cluster{"Signal Type":u16, "DC":dbl, "Amplitude":dbl, dbl, "Phase":dbl}[][]
  T12 = cluster{"Signal Type":u16, "DC":dbl, "Amplitude":dbl, dbl, "Phase":dbl}
  T13 = cluster{"Channel":u16, "Gain":u16, "Shunt Resistor":u16, "Measure":u16}[]
  T14 = cluster{"Array":dbl[], "Array 2":dbl[], "Array":dbl[], "Array 2":dbl[], "Array":dbl[], "Array 2":dbl[], "Array":dbl[], "Array 2":dbl[], "Array":dbl[], "Array 2":dbl[]}
  T15 = cluster{"Display 1":string, "Display 2":string, "Display 1":string, "Display 2":string, "Display 1":string, "Display 2":string, "Display 1":string, "Display 2":string, "Display 1":string, "Display 2":string}
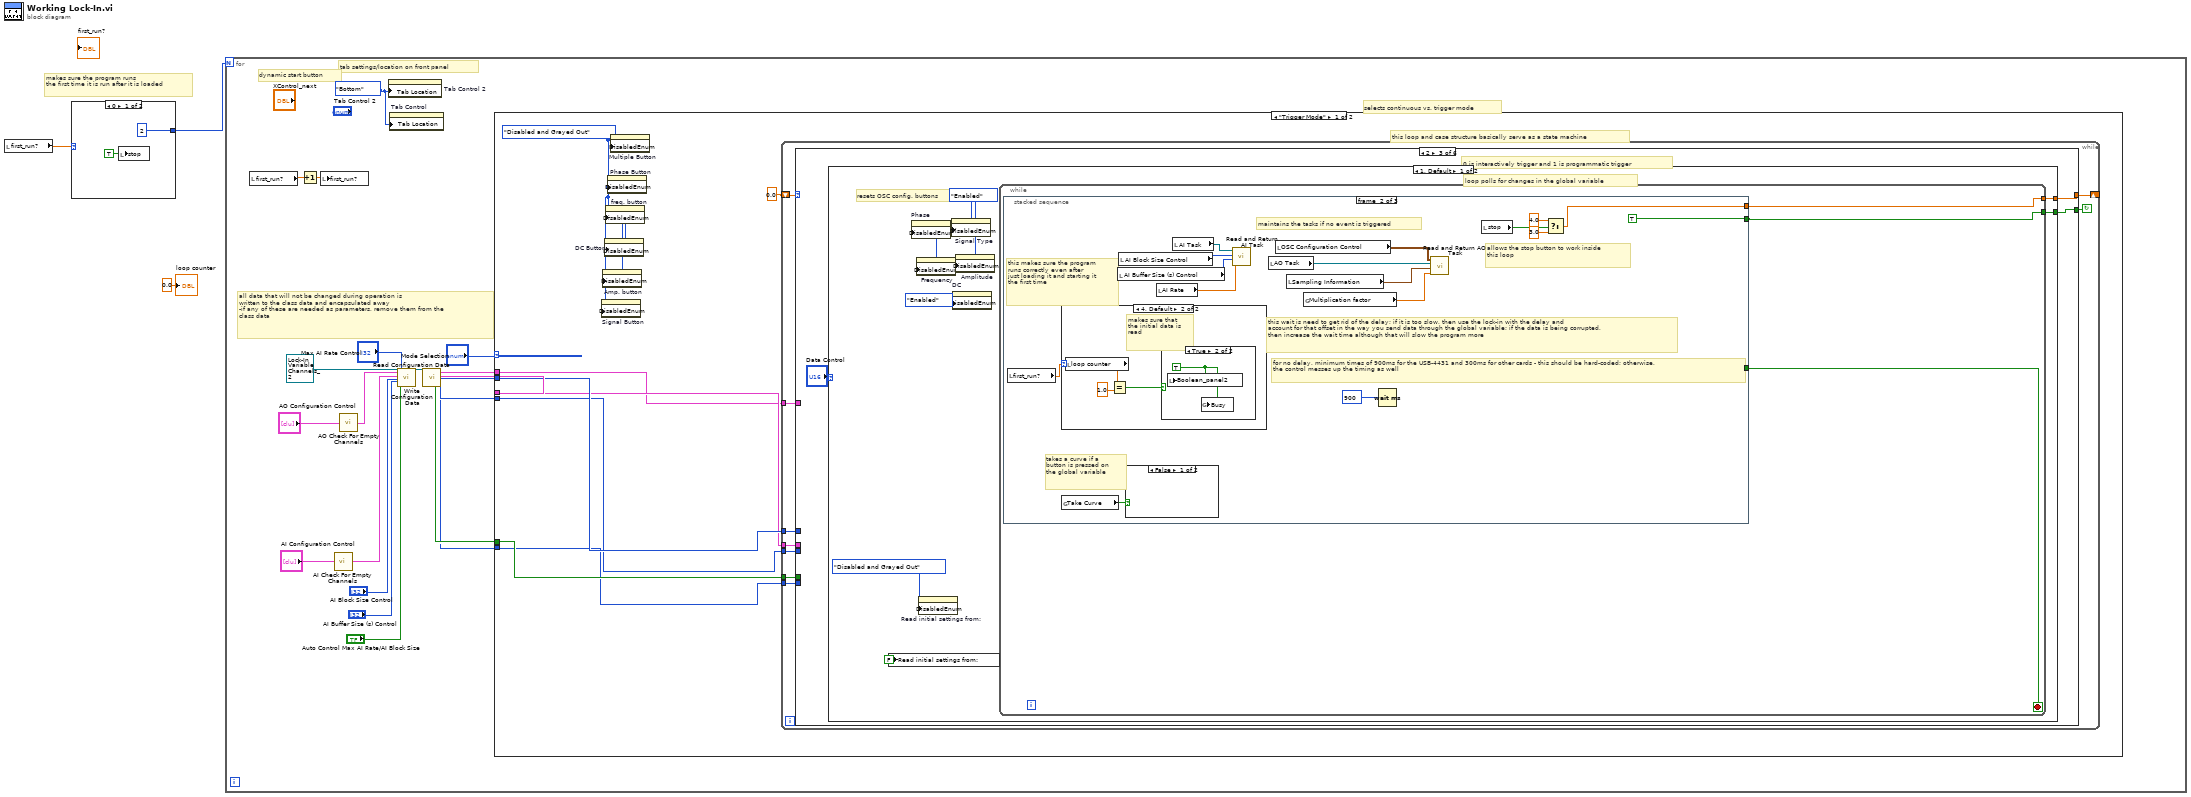
[diagram p0: block diagram]
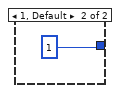
[diagram p2: hidden frame]
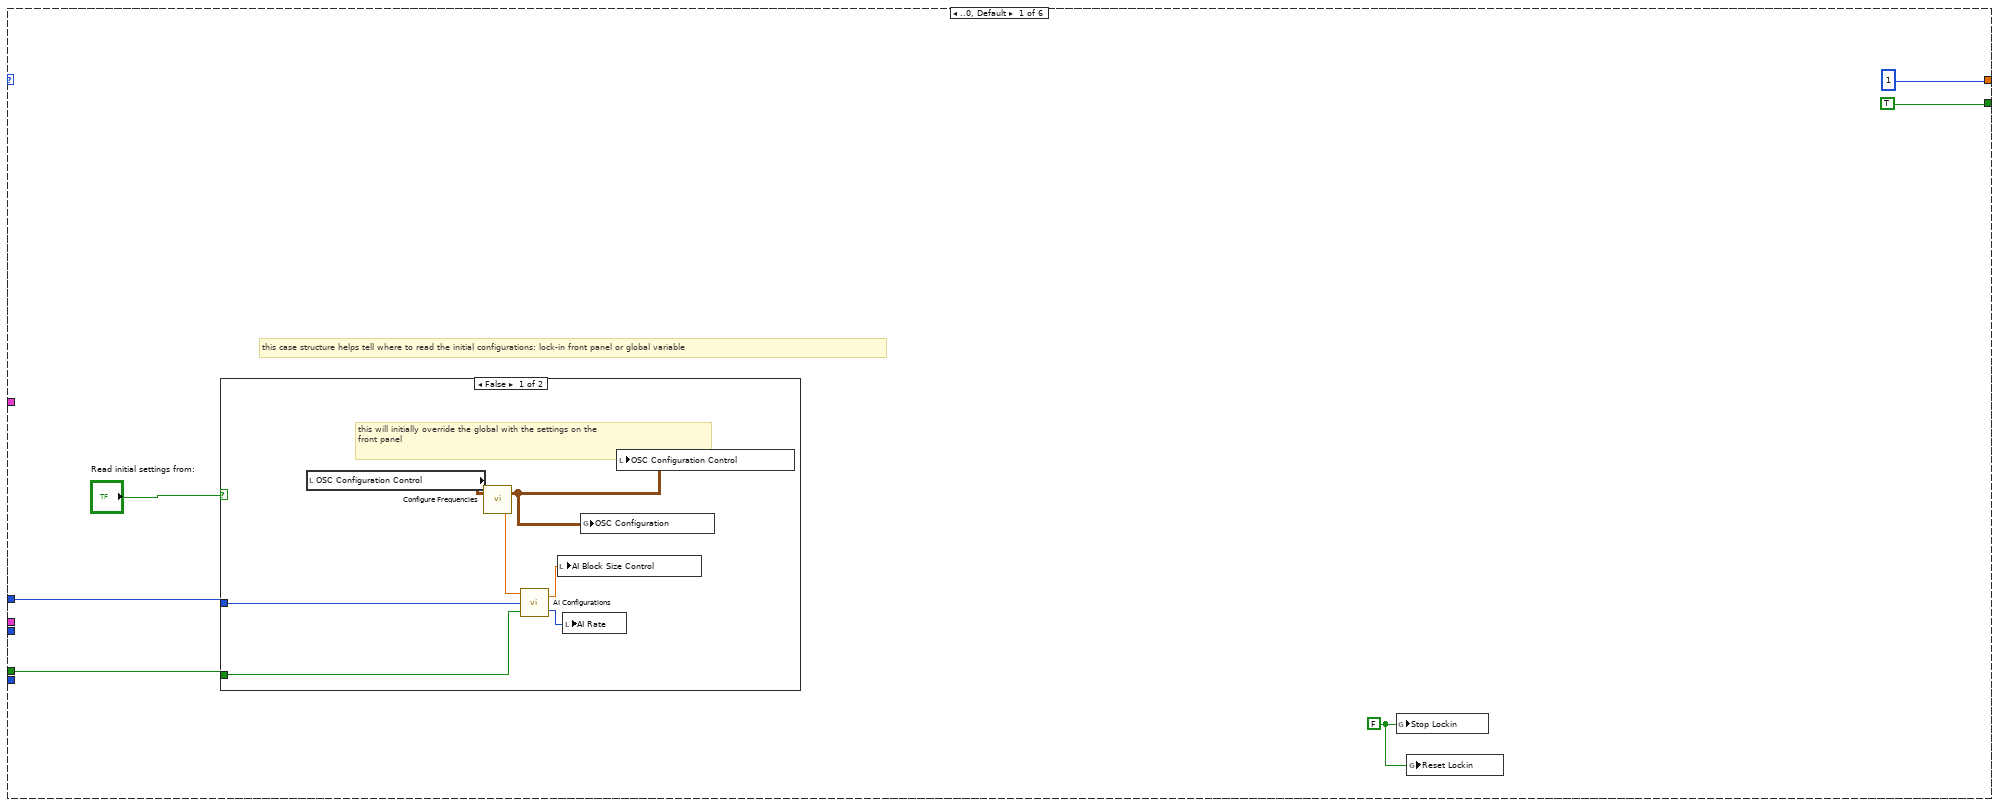
[diagram p3: hidden frame]
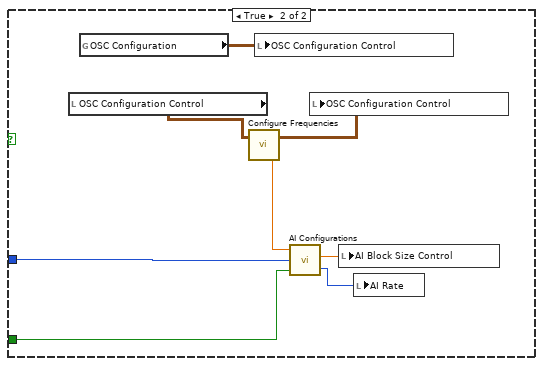
[diagram p4: hidden frame]
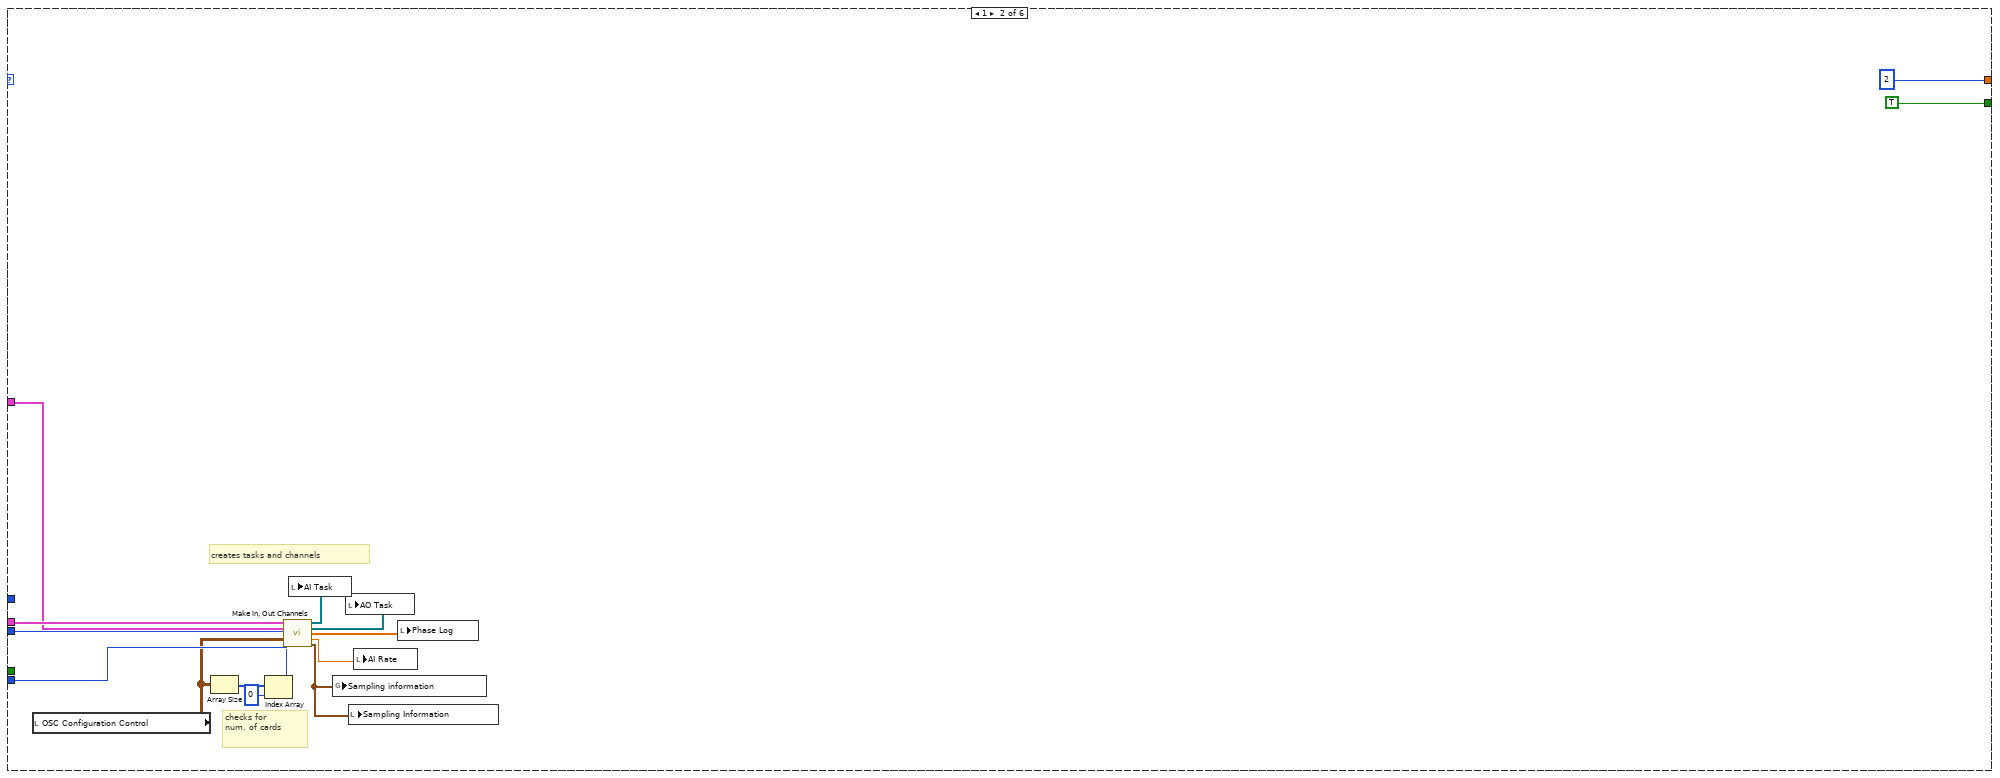
[diagram p5: hidden frame]
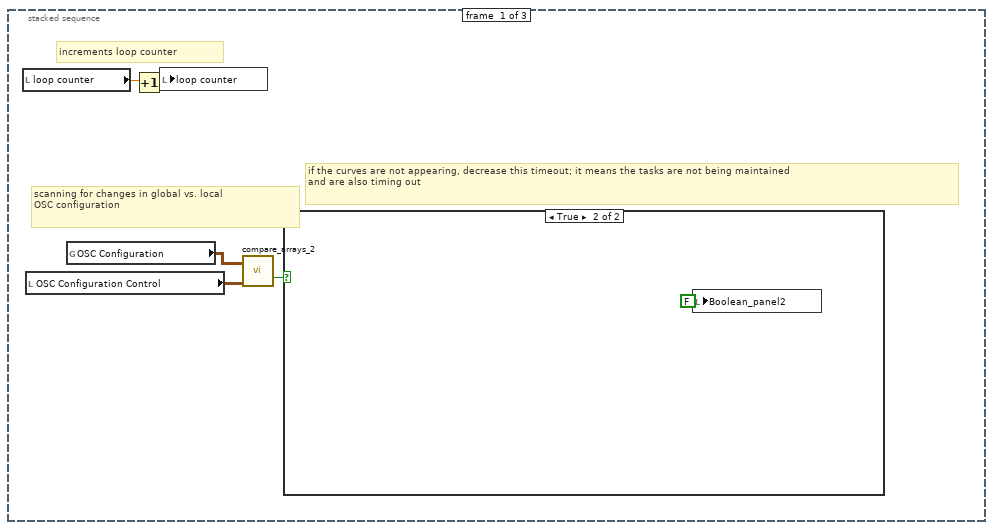
[diagram p6: hidden frame]
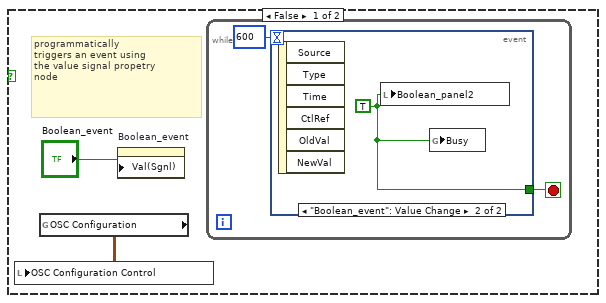
[diagram p7: hidden frame]
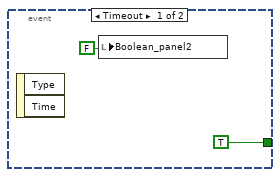
[diagram p8: hidden frame]
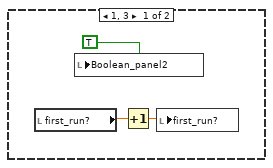
[diagram p9: hidden frame]
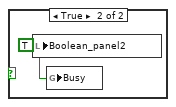
[diagram p11: hidden frame]
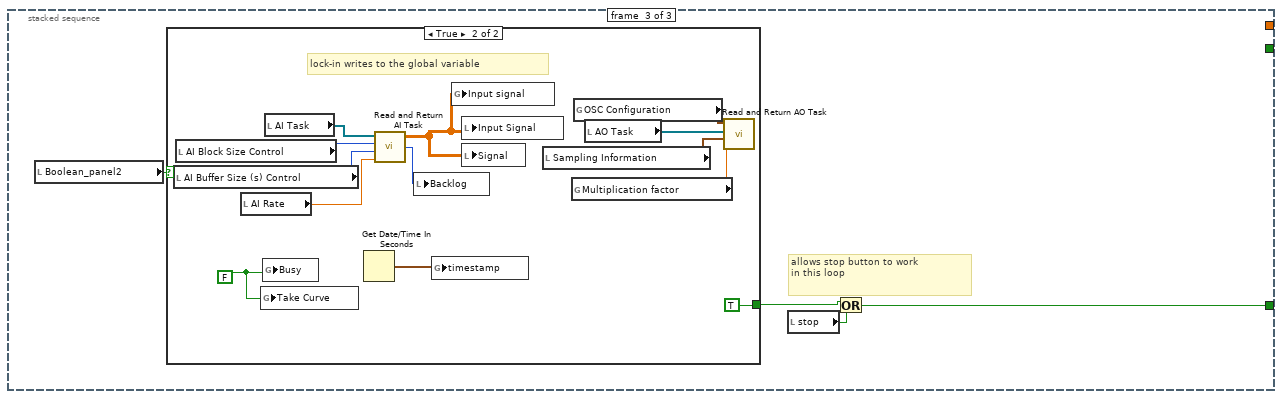
[diagram p12: hidden frame]
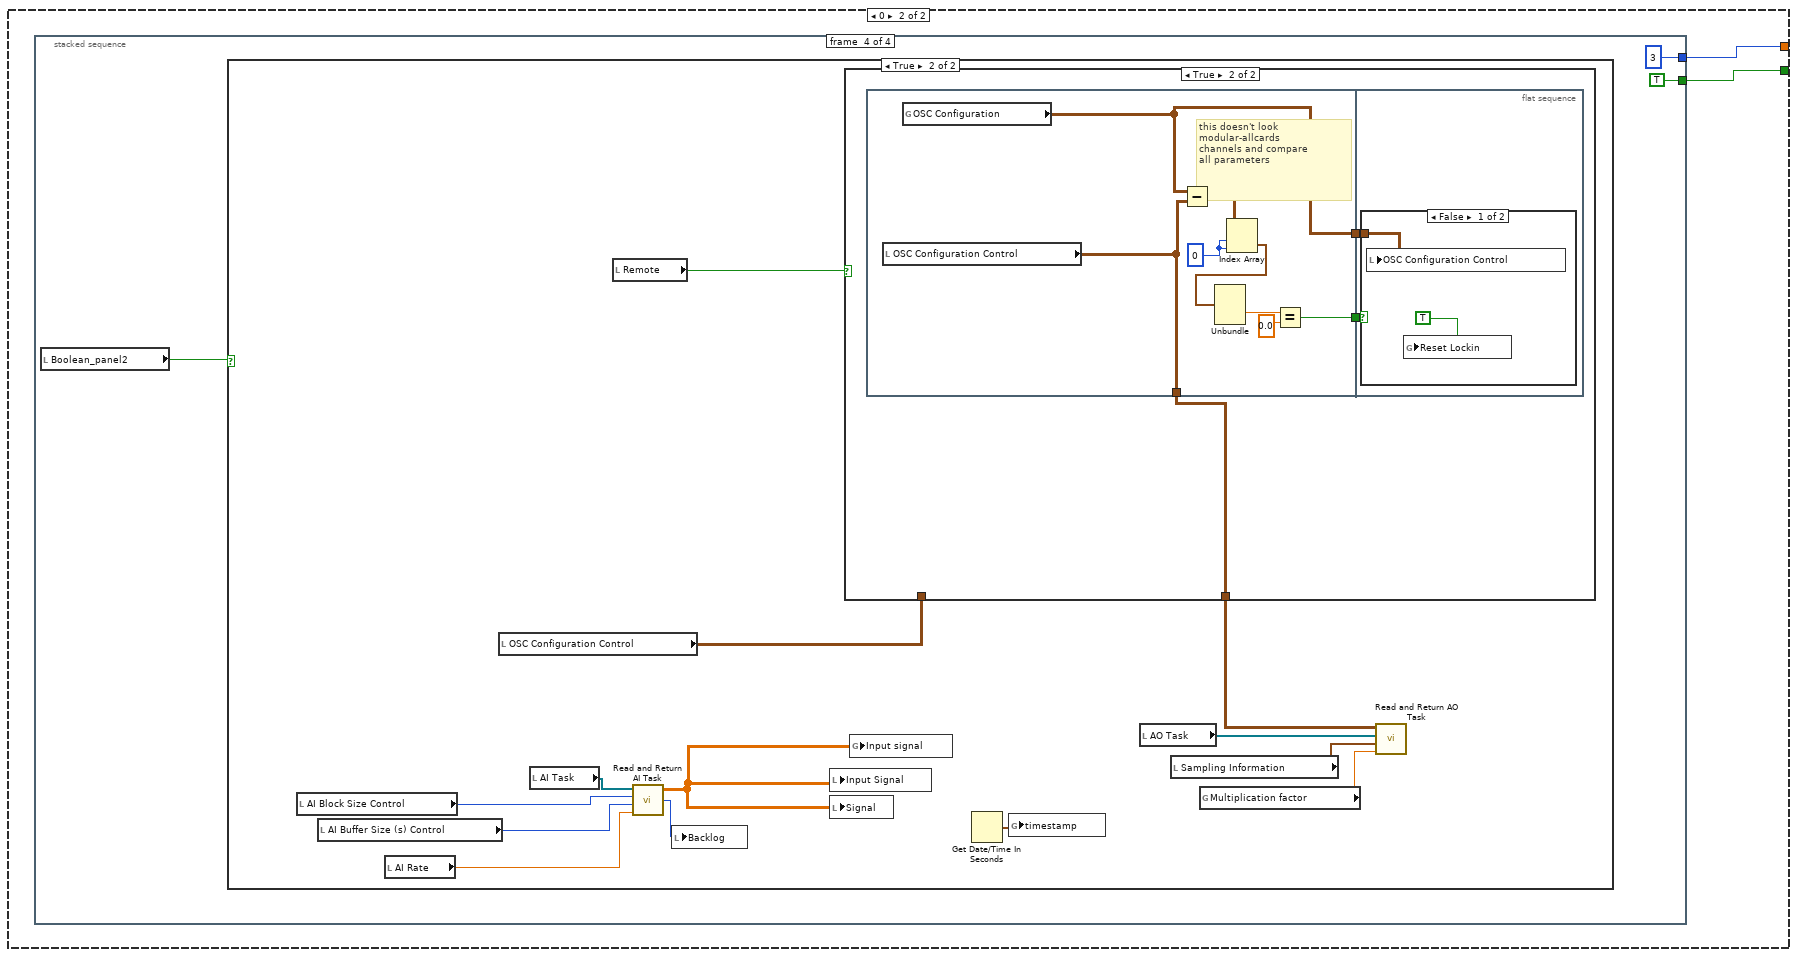
[diagram p14: hidden frame]
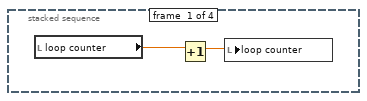
[diagram p15: hidden frame]
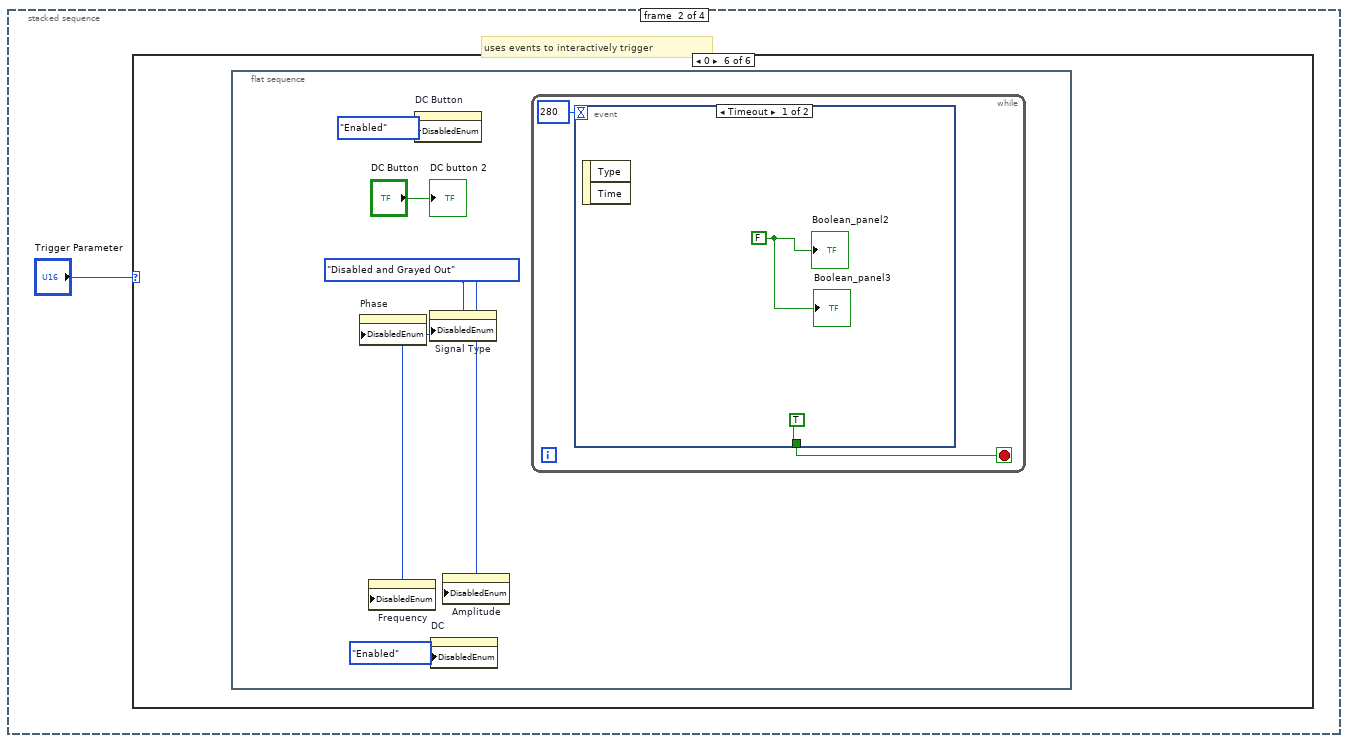
[diagram p16: hidden frame]
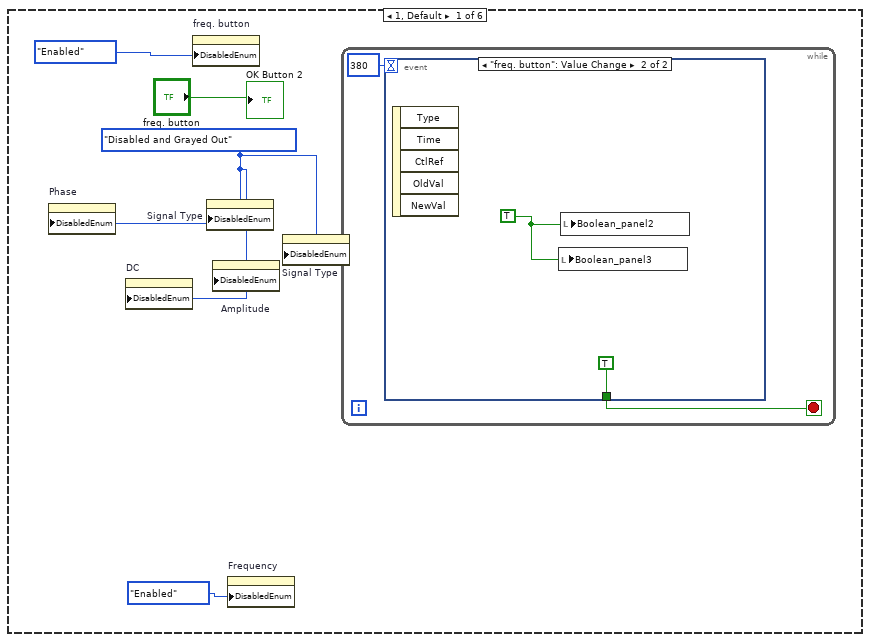
[diagram p17: hidden frame]
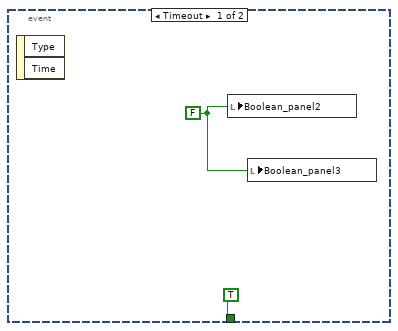
[diagram p18: hidden frame]
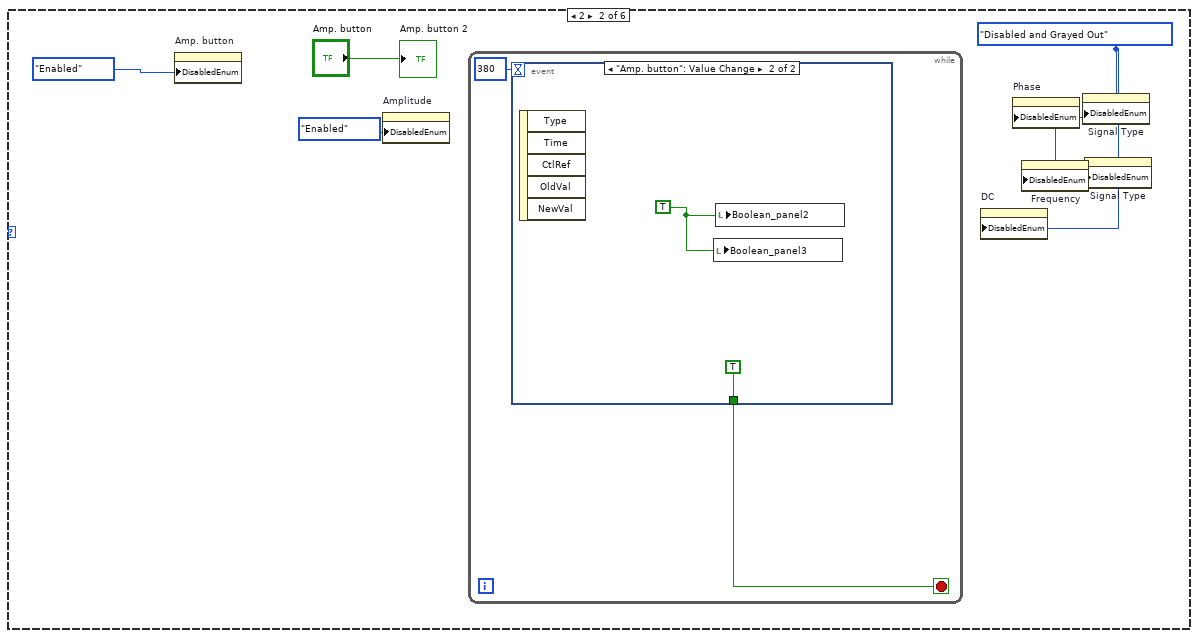
[diagram p19: hidden frame]
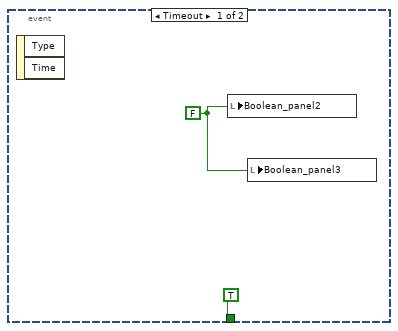
[diagram p20: hidden frame]
diagram:
  # "makes sure the program runs\nthe first time it is run after it is loaded"
  n1 = local read "first_run?"() -> (w3:dbl)
  n2 = case shown="0" w3 {
    tunnel: [2 1] -> w2
    frame 0 {
      n3 = local write "stop"(TRUE ("stop")) -> ()
    }
    frame 1, Default {
    }
  }
  n4 = for {
    N: w2 -> [_]
    w11 = enum32{"Top", "Bottom", "Left", "Right"}."Bottom" ("Tab Location")
    # "selects continuous vs. trigger mode"
    # "tab settings/location on front panel"
    # "all data that will not be changed during operation is\nwritten to the class data and encapsulated away\n-if any of these are needed as parameters, remove them from the \nclass data"
    # "dynamic start button"
    n5 = local read "first_run?"() -> (w8:dbl)
    n6 = Increment(x=w8) -> (x+1=w7:dbl)
    n7 = local write "first_run?"(w7) -> ()
    n8 = call "AI Check For Empty Channels.vi"("AI Configuration In"="AI Configuration Control") -> ("AI Configuration Out"=w18:T4)
    n9 = call "AO Check For Empty Channels.vi"("AO Configuration In"="AO Configuration Control") -> ("AO Configuration Out"=w20:T5)
    n10 = property on="Tab Control 2" class="TabCtl (strict)"("Tab Location"=w11) -> ()  [unwired: 2 in, 2 out]
    n11 = property on="Tab Control" class="TabCtl (strict)"("Tab Location"=w11) -> ()  [unwired: 2 in, 2 out]
    n12 = call-dynamic "Write Configuration Data.vi"("Lock-In Variable Channels in"=refnum<class "Lock-In Variable Channels_2.lvclass"> refnum ("Lock-In Variable Channels.lvclass"), "AO Configuration Control"=w20, "AI Configuration Control"=w18, "AI Block Size Control"="AI Block Size Control", "AI Buffer Size (s) Control"="AI Buffer Size (s) Control", "Max AI Rate Control"="Max AI Rate Control", "Auto Control Max AI Rate/AI Block Size Control"="Auto Control Max AI Rate/AI Block Size") -> ("Lock-In Variable Channels out"=w17:refnum<class "Lock-In Variable Channels_2.lvclass">)  [unwired: 19 in, 1 out]
    n13 = call-dynamic "Read Configuration Data.vi"("Lock-In Variable Channels in"=w17) -> ("Max AI Rate"=w9:i32, "Auto Control Max AI Rate/AI Block Size"=w16:bool, "AO Configuration"=w14:T5, "AI Configuration"=w15:T4, "AI Block Size"=w12:i32, "AI Buffer Size (s)"=w13:i32)  [unwired: 16 in, 5 out]
    n14 = case shown="\"Trigger Mode\"" "Mode Selection" {
      tunnel: w16 -> [w33 w357]
      tunnel: w9 -> [w34 w356]
      tunnel: w15 -> [w32 w355]
      tunnel: w14 -> [w31 w354]
      tunnel: w13 -> [w29 w353]
      tunnel: w12 -> [w30 w352]
      frame "Trigger Mode" {
        w27 = T8."Disabled and Grayed Out" ("Disabled")
        # "this loop and case structure basically serve as a state machine"
        n15 = property on="Signal Button" class="Bool"("DisabledEnum"=w27) -> ()  [unwired: 2 in, 2 out]
        n16 = property on="Amp. button" class="Bool"("DisabledEnum"=w27) -> ()  [unwired: 2 in, 2 out]
        n17 = property on="DC Button" class="Bool"("DisabledEnum"=w27) -> ()  [unwired: 2 in, 2 out]
        n18 = property on="freq. button" class="Bool"("DisabledEnum"=w27) -> ()  [unwired: 2 in, 2 out]
        n19 = property on="Phase Button" class="Bool"("DisabledEnum"=w27) -> ()  [unwired: 2 in, 2 out]
        n20 = property on="Multiple Button" class="Bool"("DisabledEnum"=w27) -> ()  [unwired: 2 in, 2 out]
        n21 = while {
          shift-right: [w43] -> _
          shift-left: 0.0 ("f") -> [w35]
          tunnel: w33 -> [w41]
          tunnel: w34 -> [w40]
          tunnel: w32 -> [w39]
          tunnel: w31 -> [w38]
          tunnel: w29 -> [w37]
          tunnel: w30 -> [w36]
          stop <- w42 continue-if-true
          n22 = case shown="2" w35 {
            tunnel: [1 2 w82 w278 w345 0.0 ("f")] -> w43
            tunnel: [TRUE TRUE w81 TRUE FALSE TRUE] -> w42
            tunnel: w41 -> [w47 _ _ _ _ _]
            tunnel: w40 -> [w46 _ _ _ _ _]
            tunnel: w39 -> [_ w79 _ _ _ _]
            tunnel: w38 -> [_ w78 _ _ _ _]
            tunnel: w37 -> [_ w71 _ _ _ _]
            tunnel: w36 -> [_ w77 _ _ _ _]
            selector: w35 -> [_ _ _ _ w345 _]
            frame ..0, Default {
              w45 = FALSE ("Stop Lockin")
              # "this case structure helps tell where to read the initial configurations: lock-in front panel or global variable"
              n23 = case shown="False" "Read initial settings from:" {
                tunnel: w47 -> [w55 w63]
                tunnel: w46 -> [w54 w62]
                frame False {
                  # "this will initially override the global with the settings on the\nfront panel"
                  n24 = local read "OSC Configuration Control"() -> (w52:T6)
                  n25 = call "Configure Frequencies.vi"("OSC Configuration In"=w52) -> ("Frequency Out"=w56:dbl, "OSC Configuation Out"=w53:T9)  [unwired: 1 in]
                  n26 = call "AI Configurations.vi"("Auto control  max AI rate/ AI block size"=w55, "Max AI Rate In"=w54, "Frequency In"=w56) -> ("AI Rate Out"=w50:i32, "AI Block Size Out"=w51:dbl)
                  n27 = local write "AI Block Size Control"(w51) -> ()
                  n28 = local write "AI Rate"(w50) -> ()
                  n29 = global write "Lock-in Globles Multiple Inputs and Outputs.vi" "OSC Configuration"(w53) -> ()
                  n30 = local write "OSC Configuration Control"(w53) -> ()
                }
                frame True {
                  n31 = local read "OSC Configuration Control"() -> (w60:T6)
                  n32 = global read "Lock-in Globles Multiple Inputs and Outputs.vi" "OSC Configuration"() -> (w59:T9)
                  n33 = call "Configure Frequencies.vi"("OSC Configuration In"=w60) -> ("Frequency Out"=w64:dbl, "OSC Configuation Out"=w61:T9)  [unwired: 1 in]
                  n34 = local write "OSC Configuration Control"(w59) -> ()
                  n35 = call "AI Configurations.vi"("Auto control  max AI rate/ AI block size"=w63, "Max AI Rate In"=w62, "Frequency In"=w64) -> ("AI Rate Out"=w57:i32, "AI Block Size Out"=w58:dbl)
                  n36 = local write "OSC Configuration Control"(w61) -> ()
                  n37 = local write "AI Block Size Control"(w58) -> ()
                  n38 = local write "AI Rate"(w57) -> ()
                }
              }
              n39 = global write "Lock-in Globles Multiple Inputs and Outputs.vi" "Stop Lockin"(w45) -> ()
              n40 = global write "Lock-in Globles Multiple Inputs and Outputs.vi" "Reset Lockin"(w45) -> ()
            }
            frame 1 {
              # "creates tasks and channels"
              # "checks for \nnum. of cards"
              n41 = local read "OSC Configuration Control"() -> (w72:T6)
              n42 = Array Size(array=w72) -> (size(s)=w74:i32[])
              n43 = Index Array(array=w74, index=0) -> (element=w65:i32)
              n44 = call "Make In, Out Channels.vi"("AI Configuration In"=w79, "AI Buffer Size (s) In"=w71, "AO Configuration Out"=w78, "Num. of Cards"=w65, "OSC Configuration In"=w72, "AI Block Size In"=w77) -> ("AI Task Out"=w70:refnum<k21>[], "AO Task Out"=w69:refnum<k21>[], "Phase Log Out"=w68:dbl[], "AI Rate Out"=w66:dbl, "Sampling Information Out"=w67:cluster{"Fs":dbl, "#s":dbl}[])  [unwired: 5 in]
              n45 = local write "AI Task"(w70) -> ()
              n46 = global write "Lock-in Globles Multiple Inputs and Outputs.vi" "Sampling information"(w67) -> ()
              n47 = local write "AO Task"(w69) -> ()
              n48 = local write "Sampling Information"(w67) -> ()
              n49 = local write "AI Rate"(w66) -> ()
              n50 = local write "Phase Log"(w68) -> ()
            }
            frame 2 {
              # "0 is interactively trigger and 1 is programmatic trigger"
              n51 = case shown="1, Default" "Data Control" {
                tunnel: [w88 w147] -> w82
                tunnel: [w87 w146] -> w81
                frame 1, Default {
                  w85 = T8."Enabled" ("Disabled")
                  # "loop polls for changes in the global variable"
                  # "resets OSC config. buttons"
                  n52 = local write "Read initial settings from:"(FALSE ("Read initial settings from:")) -> ()
                  n53 = property on="Phase" class="DigNum (strict)"("DisabledEnum"=w85) -> ()  [unwired: 2 in, 2 out]
                  n54 = property on="Frequency" class="DigNum (strict)"("DisabledEnum"=w85) -> ()  [unwired: 2 in, 2 out]
                  n55 = property on="Read initial settings from:" class="Bool (strict)"("DisabledEnum"=T8."Disabled and Grayed Out" ("Disabled")) -> ()  [unwired: 2 in, 2 out]
                  n56 = property on="Signal Type" class="Enum (strict)"("DisabledEnum"=w85) -> ()  [unwired: 2 in, 2 out]
                  n57 = property on="DC" class="DigNum (strict)"("DisabledEnum"=T8."Enabled" ("Disabled")) -> ()  [unwired: 2 in, 2 out]
                  n58 = property on="Amplitude" class="DigNum (strict)"("DisabledEnum"=w85) -> ()  [unwired: 2 in, 2 out]
                  n59 = while {
                    tunnel: [w91] -> w88
                    tunnel: [w90] -> w87
                    stop <- w89 stop-if-true
                    n60 = stacked-sequence {
                      tunnel: [_ w116 _] -> w91
                      tunnel: [_ TRUE _] -> w90
                      tunnel: [_ _ w129] -> w89
                      frame #0 {
                        # "increments loop counter"
                        # "if the curves are not appearing, decrease this timeout; it means the tasks are not being maintained\nand are also timing out"
                        # "scanning for changes in global vs. local \nOSC configuration"
                        n61 = local read "loop counter"() -> (w96:dbl)
                        n62 = local read "OSC Configuration Control"() -> (w93:T6)
                        n63 = global read "Lock-in Globles Multiple Inputs and Outputs.vi" "OSC Configuration"() -> (w94:T9)
                        n64 = Increment(x=w96) -> (x+1=w95:dbl)
                        n65 = local write "loop counter"(w95) -> ()
                        n66 = call "compare_arrays_2.vi"("OSC Configuration Control"=w93, "OSC Global Variable"=w94) -> ("are the same?"=w92:bool)
                        n67 = case shown="True" w92 {
                          frame False {
                            # "programmatically\ntriggers an event using\nthe value signal propetry\nnode"
                            n68 = global read "Lock-in Globles Multiple Inputs and Outputs.vi" "OSC Configuration"() -> (w97:T9)
                            n69 = local write "OSC Configuration Control"(w97) -> ()
                            n70 = property on="Boolean_event" class="Bool (strict)"("Val(Sgnl)"="Boolean_event") -> ()  [unwired: 2 in, 2 out]
                            n71 = while {
                              stop <- w99 stop-if-true
                              n72 = event shown="[1] \"Boolean_event\": Value Change" {
                                selector: _ -> [_ _]
                                dyn-events: _ -> [_ _]
                                timeout: 600 -> [_ _]
                                tunnel: [TRUE w103] -> w99
                                event Timeout {
                                n73 = event-data() -> ()  [unwired: 1 in, 2 out]
                                n74 = local write "Boolean_panel2"(FALSE) -> ()
                                }
                                event "Boolean_event": Value Change {
                                w103 = TRUE
                                n75 = event-data() -> ()  [unwired: 1 in, 6 out]
                                n76 = local write "Boolean_panel2"(w103) -> ()
                                n77 = global write "Lock-in Globles Multiple Inputs and Outputs.vi" "Busy"(w103) -> ()
                                }
                              }
                            }
                          }
                          frame True {
                            n78 = local write "Boolean_panel2"(FALSE ("Boolean_panel2")) -> ()
                          }
                        }
                      }
                      frame #1 {
                        # "this makes sure the program\nruns correctly even after\njust loading it and starting it\nthe first time"
                        # "for no delay, minimum times of 900ms for the USB-4431 and 300ms for other cards - this should be hard-coded; otherwise,\nthe control messes up the timing as well"
                        # "this wait is need to get rid of the delay; if it is too slow, then use the lock-in with the delay and\naccount for that offset in the way you send data through the global variable; if the data is being corrupted,\nthen increase the wait time although that will slow the program more"
                        # "takes a curve if a \nbutton is pressed on\nthe global variable"
                        # "maintains the tasks if no event is triggered"
                        # "allows the stop button to work inside\nthis loop"
                        n79 = local read "first_run?"() -> (w105:dbl)
                        n80 = global read "Lock-in Globles Multiple Inputs and Outputs.vi" "Take Curve"() -> (w107:bool)
                        n81 = case shown="4, Default" w105 {
                          frame 1, 3 {
                            n82 = local read "first_run?"() -> (w122:dbl)
                            n83 = local write "Boolean_panel2"(TRUE) -> ()
                            n84 = Increment(x=w122) -> (x+1=w121:dbl)
                            n85 = local write "first_run?"(w121) -> ()
                          }
                          frame 4, Default {
                            # "makes sure that\nthe initial data is\nread"
                            n86 = local read "loop counter"() -> (w126:dbl)
                            n87 = Equal?(x=w126, y=1.0) -> (x = y?=w124:bool)
                            n88 = case shown="True" w124 {
                              frame False {
                              }
                              frame True {
                                w127 = TRUE
                                n89 = local write "Boolean_panel2"(w127) -> ()
                                n90 = global write "Lock-in Globles Multiple Inputs and Outputs.vi" "Busy"(w127) -> ()
                              }
                            }
                          }
                        }
                        n91 = local read "AI Buffer Size (s) Control"() -> (w115:i32)
                        n92 = local read "AI Block Size Control"() -> (w114:i32)
                        n93 = case shown="False" w107 {
                          frame False {
                          }
                          frame True {
                            w128 = TRUE
                            n94 = local write "Boolean_panel2"(w128) -> ()
                            n95 = global write "Lock-in Globles Multiple Inputs and Outputs.vi" "Busy"(w128) -> ()
                          }
                        }
                        n96 = local read "AI Rate"() -> (w112:dbl)
                        n97 = local read "AI Task"() -> (w113:refnum<k21>[])
                        n98 = call "Read and Return AI Task.vi"("AI Task In"=w113, "AI Block Size In"=w114, "AI Buffer Size (s) In"=w115, "AI Rate In"=w112) -> ()  [unwired: 2 in, 2 out]
                        n99 = local read "AO Task"() -> (w110:refnum<k21>[])
                        n100 = local read "OSC Configuration Control"() -> (w108:T6)
                        n101 = local read "Sampling Information"() -> (w109:cluster{"Fs":dbl, "#s":dbl}[])
                        n102 = global read "Lock-in Globles Multiple Inputs and Outputs.vi" "Multiplication factor"() -> (w111:dbl)
                        n103 = Wait (ms)(milliseconds to wait=u32 900) -> ()  [unwired: 1 out]
                        n104 = call "Read and Return AO Task.vi"("OSC Configuration In"=w108, "AO Task In"=w110, "Sampling Information In"=w109, "Multiplication Factor In"=w111) -> ()  [unwired: 2 in]
                        n105 = local read "stop"() -> (w119:bool)
                        n106 = Select(t=4.0, s=w119, f=3.0) -> (s? t:f=w116:dbl)
                      }
                      frame #2 {
                        # "allows stop button to work\nin this loop"
                        n107 = local read "Boolean_panel2"() -> (w132:bool)
                        n108 = case shown="True" w132 {
                          tunnel: [_ TRUE] -> w131
                          frame False {
                          }
                          frame True {
                            w133 = FALSE ("Busy")
                            # "lock-in writes to the global variable"
                            n109 = local read "AI Buffer Size (s) Control"() -> (w141:i32)
                            n110 = local read "AI Block Size Control"() -> (w142:i32)
                            n111 = local read "AI Rate"() -> (w140:dbl)
                            n112 = global write "Lock-in Globles Multiple Inputs and Outputs.vi" "Take Curve"(w133) -> ()
                            n113 = global write "Lock-in Globles Multiple Inputs and Outputs.vi" "Busy"(w133) -> ()
                            n114 = local read "AI Task"() -> (w143:refnum<k21>[])
                            n115 = Get Date/Time In Seconds() -> (seconds since 1Jan1904=w144:timestamp)
                            n116 = call "Read and Return AI Task.vi"("AI Task In"=w143, "AI Block Size In"=w142, "AI Buffer Size (s) In"=w141, "AI Rate In"=w140) -> ("Input Signal Out"=w138:dbl[][], "Backlog Out"=w139:u8)  [unwired: 2 in]
                            n117 = local write "Backlog"(w139) -> ()
                            n118 = global write "Lock-in Globles Multiple Inputs and Outputs.vi" "timestamp"(w144) -> ()
                            n119 = global write "Lock-in Globles Multiple Inputs and Outputs.vi" "Input signal"(w138) -> ()
                            n120 = local write "Input Signal"(w138) -> ()
                            n121 = local write "Signal"(w138) -> ()
                            n122 = local read "Sampling Information"() -> (w135:cluster{"Fs":dbl, "#s":dbl}[])
                            n123 = global read "Lock-in Globles Multiple Inputs and Outputs.vi" "Multiplication factor"() -> (w137:dbl)
                            n124 = global read "Lock-in Globles Multiple Inputs and Outputs.vi" "OSC Configuration"() -> (w134:T9)
                            n125 = local read "AO Task"() -> (w136:refnum<k21>[])
                            n126 = call "Read and Return AO Task.vi"("OSC Configuration In"=w134, "AO Task In"=w136, "Sampling Information In"=w135, "Multiplication Factor In"=w137) -> ()  [unwired: 2 in]
                          }
                        }
                        n127 = local read "stop"() -> (w130:bool)
                        n128 = Or(x=w131, y=w130) -> (x .or. y?=w129:bool)
                      }
                    }
                  }
                }
                frame 0 {
                  n129 = stacked-sequence {
                    tunnel: [_ _ _ 3] -> w147
                    tunnel: [_ _ _ TRUE] -> w146
                    frame #0 {
                      n130 = local read "loop counter"() -> (w149:dbl)
                      n131 = Increment(x=w149) -> (x+1=w148:dbl)
                      n132 = local write "loop counter"(w148) -> ()
                    }
                    frame #1 {
                      # "uses events to interactively trigger"
                      n133 = case shown="0" "Trigger Parameter" {
                        frame 1, Default {
                          w151 = T8."Disabled and Grayed Out" ("Disabled")
                          n134 = property on="Phase" class="DigNum (strict)"("DisabledEnum"=w151) -> ()  [unwired: 2 in, 2 out]
                          n135 = property on="DC" class="DigNum (strict)"("DisabledEnum"=w151) -> ()  [unwired: 2 in, 2 out]
                          n136 = property on="freq. button" class="Bool"("DisabledEnum"=T8."Enabled" ("Disabled")) -> ()  [unwired: 2 in, 2 out]
                          n137 = property on="Signal Type" class="Enum (strict)"("DisabledEnum"=w151) -> ()  [unwired: 2 in, 2 out]
                          n138 = property on="Amplitude" class="DigNum (strict)"("DisabledEnum"=w151) -> ()  [unwired: 2 in, 2 out]
                          n139 = property on="Frequency" class="DigNum (strict)"("DisabledEnum"=T8."Enabled" ("Disabled")) -> ()  [unwired: 2 in, 2 out]
                          n140 = property on="Signal Type" class="Enum (strict)"("DisabledEnum"=w151) -> ()  [unwired: 2 in, 2 out]
                          n141 = while {
                            stop <- w155 stop-if-true
                            n142 = event shown="[1] \"freq. button\": Value Change" {
                              selector: _ -> [_ _]
                              dyn-events: _ -> [_ _]
                              timeout: 380 -> [_ _]
                              tunnel: [TRUE ("Boolean_panel2") TRUE] -> w155
                              event Timeout {
                                w157 = FALSE ("Boolean_panel2")
                                n143 = event-data() -> ()  [unwired: 1 in, 2 out]
                                n144 = local write "Boolean_panel2"(w157) -> ()
                                n145 = local write "Boolean_panel3"(w157) -> ()
                              }
                              event "freq. button": Value Change {
                                w159 = TRUE
                                n146 = event-data() -> ()  [unwired: 1 in, 5 out]
                                n147 = local write "Boolean_panel3"(w159) -> ()
                                n148 = local write "Boolean_panel2"(w159) -> ()
                              }
                            }
                          }
                          "OK Button 2" <- "freq. button"
                        }
                        frame 2 {
                          w162 = T8."Disabled and Grayed Out" ("Disabled")
                          n149 = property on="Amp. button" class="Bool"("DisabledEnum"=T8."Enabled" ("Disabled")) -> ()  [unwired: 2 in, 2 out]
                          n150 = property on="Amplitude" class="DigNum (strict)"("DisabledEnum"=T8."Enabled" ("Disabled")) -> ()  [unwired: 2 in, 2 out]
                          n151 = while {
                            stop <- w165 stop-if-true
                            n152 = event shown="[1] \"Amp. button\": Value Change" {
                              selector: _ -> [_ _]
                              dyn-events: _ -> [_ _]
                              timeout: 380 -> [_ _]
                              tunnel: [TRUE ("Boolean_panel2") TRUE] -> w165
                              event Timeout {
                                w167 = FALSE ("Boolean_panel2")
                                n153 = event-data() -> ()  [unwired: 1 in, 2 out]
                                n154 = local write "Boolean_panel2"(w167) -> ()
                                n155 = local write "Boolean_panel3"(w167) -> ()
                              }
                              event "Amp. button": Value Change {
                                w169 = TRUE
                                n156 = event-data() -> ()  [unwired: 1 in, 5 out]
                                n157 = local write "Boolean_panel3"(w169) -> ()
                                n158 = local write "Boolean_panel2"(w169) -> ()
                              }
                            }
                          }
                          n159 = property on="DC" class="DigNum (strict)"("DisabledEnum"=w162) -> ()  [unwired: 2 in, 2 out]
                          n160 = property on="Phase" class="DigNum (strict)"("DisabledEnum"=w162) -> ()  [unwired: 2 in, 2 out]
                          n161 = property on="Frequency" class="DigNum (strict)"("DisabledEnum"=w162) -> ()  [unwired: 2 in, 2 out]
                          n162 = property on="Signal Type" class="Enum (strict)"("DisabledEnum"=w162) -> ()  [unwired: 2 in, 2 out]
                          n163 = property on="Signal Type" class="Enum (strict)"("DisabledEnum"=w162) -> ()  [unwired: 2 in, 2 out]
                          "Amp. button 2" <- "Amp. button"
                        }
                        frame 3 {
                          w171 = T8."Disabled and Grayed Out" ("Disabled")
                          n164 = property on="DC" class="DigNum (strict)"("DisabledEnum"=w171) -> ()  [unwired: 2 in, 2 out]
                          n165 = property on="Phase" class="DigNum (strict)"("DisabledEnum"=w171) -> ()  [unwired: 2 in, 2 out]
                          n166 = property on="Frequency" class="DigNum (strict)"("DisabledEnum"=w171) -> ()  [unwired: 2 in, 2 out]
                          n167 = property on="Signal Button" class="Bool"("DisabledEnum"=T8."Enabled" ("Disabled")) -> ()  [unwired: 2 in, 2 out]
                          n168 = property on="Signal Type" class="Enum (strict)"("DisabledEnum"=w171) -> ()  [unwired: 2 in, 2 out]
                          n169 = property on="Signal Type" class="Enum (strict)"("DisabledEnum"=T8."Enabled" ("Disabled")) -> ()  [unwired: 2 in, 2 out]
                          n170 = property on="Amplitude" class="DigNum (strict)"("DisabledEnum"=w171) -> ()  [unwired: 2 in, 2 out]
                          n171 = while {
                            stop <- w175 stop-if-true
                            n172 = event shown="[1] \"Signal Button\": Value Change" {
                              selector: _ -> [_ _]
                              dyn-events: _ -> [_ _]
                              timeout: 380 -> [_ _]
                              tunnel: [TRUE ("Boolean_panel2") TRUE] -> w175
                              event Timeout {
                                w177 = FALSE ("Boolean_panel2")
                                n173 = event-data() -> ()  [unwired: 1 in, 2 out]
                                n174 = local write "Boolean_panel2"(w177) -> ()
                                n175 = local write "Boolean_panel3"(w177) -> ()
                              }
                              event "Signal Button": Value Change {
                                w179 = TRUE
                                n176 = event-data() -> ()  [unwired: 1 in, 5 out]
                                n177 = local write "Boolean_panel3"(w179) -> ()
                                n178 = local write "Boolean_panel2"(w179) -> ()
                              }
                            }
                          }
                          "Signal indicator" <- "Signal Button"
                        }
                        frame 4 {
                          w181 = T8."Disabled and Grayed Out" ("Disabled")
                          n179 = property on="DC" class="DigNum (strict)"("DisabledEnum"=w181) -> ()  [unwired: 2 in, 2 out]
                          n180 = property on="Signal Type" class="Enum (strict)"("DisabledEnum"=w181) -> ()  [unwired: 2 in, 2 out]
                          n181 = property on="Frequency" class="DigNum (strict)"("DisabledEnum"=w181) -> ()  [unwired: 2 in, 2 out]
                          n182 = property on="Phase Button" class="Bool"("DisabledEnum"=T8."Enabled" ("Disabled")) -> ()  [unwired: 2 in, 2 out]
                          n183 = property on="Signal Type" class="Enum (strict)"("DisabledEnum"=w181) -> ()  [unwired: 2 in, 2 out]
                          n184 = property on="Amplitude" class="DigNum (strict)"("DisabledEnum"=w181) -> ()  [unwired: 2 in, 2 out]
                          n185 = property on="Phase" class="DigNum (strict)"("DisabledEnum"=T8."Enabled" ("Disabled")) -> ()  [unwired: 2 in, 2 out]
                          n186 = while {
                            stop <- w185 stop-if-true
                            n187 = event shown="[1] \"Phase Button\": Value Change" {
                              selector: _ -> [_ _]
                              dyn-events: _ -> [_ _]
                              timeout: 380 -> [_ _]
                              tunnel: [TRUE ("Boolean_panel2") TRUE] -> w185
                              event Timeout {
                                w187 = FALSE ("Boolean_panel2")
                                n188 = event-data() -> ()  [unwired: 1 in, 2 out]
                                n189 = local write "Boolean_panel2"(w187) -> ()
                                n190 = local write "Boolean_panel3"(w187) -> ()
                              }
                              event "Phase Button": Value Change {
                                w189 = TRUE
                                n191 = event-data() -> ()  [unwired: 1 in, 5 out]
                                n192 = local write "Boolean_panel3"(w189) -> ()
                                n193 = local write "Boolean_panel2"(w189) -> ()
                              }
                            }
                          }
                          "Phase indicator" <- "Phase Button"
                        }
                        frame 5 {
                          w191 = T8."Enabled" ("Disabled")
                          n194 = property on="Phase" class="DigNum (strict)"("DisabledEnum"=w191) -> ()  [unwired: 2 in, 2 out]
                          n195 = property on="Frequency" class="DigNum (strict)"("DisabledEnum"=w191) -> ()  [unwired: 2 in, 2 out]
                          n196 = property on="Signal Type" class="Enum (strict)"("DisabledEnum"=w191) -> ()  [unwired: 2 in, 2 out]
                          n197 = property on="Amplitude" class="DigNum (strict)"("DisabledEnum"=w191) -> ()  [unwired: 2 in, 2 out]
                          n198 = property on="Multiple Button" class="Bool"("DisabledEnum"=T8."Enabled" ("Disabled")) -> ()  [unwired: 2 in, 2 out]
                          n199 = property on="Signal Type" class="Enum (strict)"("DisabledEnum"=w191) -> ()  [unwired: 2 in, 2 out]
                          n200 = while {
                            stop <- w194 stop-if-true
                            n201 = event shown="[1] \"Multiple Button\": Value Change" {
                              selector: _ -> [_ _]
                              dyn-events: _ -> [_ _]
                              timeout: 380 -> [_ _]
                              tunnel: [TRUE ("Boolean_panel2") TRUE] -> w194
                              event Timeout {
                                w196 = FALSE ("Boolean_panel2")
                                n202 = event-data() -> ()  [unwired: 1 in, 2 out]
                                n203 = local write "Boolean_panel2"(w196) -> ()
                                n204 = local write "Boolean_panel3"(w196) -> ()
                              }
                              event "Multiple Button": Value Change {
                                w198 = TRUE
                                n205 = event-data() -> ()  [unwired: 1 in, 5 out]
                                n206 = local write "Boolean_panel3"(w198) -> ()
                                n207 = local write "Boolean_panel2"(w198) -> ()
                              }
                            }
                          }
                          "Multiple Indicator" <- "Multiple Button"
                        }
                        frame 0 {
                          n208 = flat-sequence {
                            frame #0 {
                              w201 = T8."Disabled and Grayed Out" ("Disabled")
                              n209 = property on="Phase" class="DigNum (strict)"("DisabledEnum"=w201) -> ()  [unwired: 2 in, 2 out]
                              n210 = property on="Frequency" class="DigNum (strict)"("DisabledEnum"=w201) -> ()  [unwired: 2 in, 2 out]
                              n211 = property on="DC Button" class="Bool"("DisabledEnum"=T8."Enabled" ("Disabled")) -> ()  [unwired: 2 in, 2 out]
                              n212 = property on="Signal Type" class="Enum (strict)"("DisabledEnum"=w201) -> ()  [unwired: 2 in, 2 out]
                              n213 = property on="DC" class="DigNum (strict)"("DisabledEnum"=T8."Enabled" ("Disabled")) -> ()  [unwired: 2 in, 2 out]
                              n214 = property on="Amplitude" class="DigNum (strict)"("DisabledEnum"=w201) -> ()  [unwired: 2 in, 2 out]
                              n215 = while {
                                stop <- w204 stop-if-true
                                n216 = event shown="[0] Timeout" {
                                selector: _ -> [_ _]
                                dyn-events: _ -> [_ _]
                                timeout: 280 -> [_ _]
                                tunnel: [TRUE ("Boolean_panel2") TRUE] -> w204
                                event Timeout {
                                w207 = FALSE ("Boolean_panel2")
                                n217 = event-data() -> ()  [unwired: 1 in, 2 out]
                                "Boolean_panel2" <- w207
                                "Boolean_panel3" <- w207
                                }
                                event "DC Button": Value Change {
                                w209 = TRUE
                                n218 = event-data() -> ()  [unwired: 1 in, 5 out]
                                n219 = local write "Boolean_panel2"(w209) -> ()
                                n220 = local write "Boolean_panel3"(w209) -> ()
                                }
                                }
                              }
                              "DC button 2" <- "DC Button"
                            }
                          }
                        }
                      }
                    }
                    frame #2 {
                      # "reads initially entered data"
                      n221 = local read "loop counter"() -> (w212:dbl)
                      n222 = Equal?(x=w212, y=1.0) -> (x = y?=w210:bool)
                      n223 = case shown="True" w210 {
                        frame False {
                        }
                        frame True {
                          w213 = TRUE
                          n224 = local write "Boolean_panel3"(w213) -> ()
                          n225 = local write "Boolean_panel2"(w213) -> ()
                        }
                      }
                    }
                    frame #3 {
                      n226 = local read "Boolean_panel2"() -> (w214:bool)
                      n227 = case shown="True" w214 {
                        frame False {
                          # "maintains the tasks if no event triggered"
                          n228 = local read "AI Buffer Size (s) Control"() -> (w224:i32)
                          n229 = local read "AI Block Size Control"() -> (w223:i32)
                          n230 = local read "AI Rate"() -> (w221:dbl)
                          n231 = local read "AI Task"() -> (w222:refnum<k21>[])
                          n232 = call "Read and Return AI Task.vi"("AI Task In"=w222, "AI Block Size In"=w223, "AI Buffer Size (s) In"=w224, "AI Rate In"=w221) -> ()  [unwired: 2 in, 2 out]
                          n233 = local read "AO Task"() -> (w219:refnum<k21>[])
                          n234 = local read "OSC Configuration Control"() -> (w217:T6)
                          n235 = local read "Sampling Information"() -> (w218:cluster{"Fs":dbl, "#s":dbl}[])
                          n236 = global read "Lock-in Globles Multiple Inputs and Outputs.vi" "Multiplication factor"() -> (w220:dbl)
                          n237 = call "Read and Return AO Task.vi"("OSC Configuration In"=w217, "AO Task In"=w219, "Sampling Information In"=w218, "Multiplication Factor In"=w220) -> ()  [unwired: 2 in]
                        }
                        frame True {
                          n238 = local read "AI Block Size Control"() -> (w235:i32)
                          n239 = local read "AI Buffer Size (s) Control"() -> (w234:i32)
                          n240 = local read "AI Rate"() -> (w233:dbl)
                          n241 = local read "OSC Configuration Control"() -> (w226:T6)
                          n242 = local read "AI Task"() -> (w236:refnum<k21>[])
                          n243 = local read "Remote"() -> (w227:bool)
                          n244 = call "Read and Return AI Task.vi"("AI Task In"=w236, "AI Block Size In"=w235, "AI Buffer Size (s) In"=w234, "AI Rate In"=w233) -> ("Input Signal Out"=w225:dbl[][], "Backlog Out"=w228:u8)  [unwired: 2 in]
                          n245 = local write "Backlog"(w228) -> ()
                          n246 = local write "Input Signal"(w225) -> ()
                          n247 = local write "Signal"(w225) -> ()
                          n248 = case shown="True" w227 {
                            tunnel: [w239 w262] -> w232
                            tunnel: w226 -> [w238 _]
                            frame False {
                              n249 = Index Array(array=w238, index (row)=0, index (col)=0 ("disabled index (col)")) -> (element=w243:T10)
                              n250 = Unbundle By Name(w243) -> ("Frequency"=w242:dbl)
                              n251 = for {
                                tunnel: w242 -> [w248]
                                tunnel: w238 -> [w247] mode=indexing
                                tunnel: [w246] -> w239 mode=indexing
                                i -> [w245]
                                n252 = Equal To 0?(x=w245) -> (x = 0?=w244:bool)
                                n253 = for {
                                tunnel: w247 -> [w255] mode=indexing
                                tunnel: w248 -> [w254]
                                tunnel: [w253] -> w246 mode=indexing
                                tunnel: w244 -> [w249]
                                i -> [w251]
                                n254 = Equal To 0?(x=w251) -> (x = 0?=w250:bool)
                                n255 = And(x=w250, y=w249) -> (x .and. y?=w252:bool)
                                n256 = case shown="False" w252 {
                                tunnel: w255 -> [w258 w259]
                                tunnel: w254 -> [w257 _]
                                tunnel: [w256 w259] -> w253
                                frame False {
                                n257 = Bundle By Name(cluster=w258, "Frequency"=w257) -> (w256:T10)
                                }
                                frame True {
                                }
                                }
                                }
                              }
                              n258 = local write "OSC Configuration Control"(w239) -> ()
                              n259 = global write "Lock-in Globles Multiple Inputs and Outputs.vi" "OSC Configuration"(w239) -> ()
                            }
                            frame True {
                              n260 = flat-sequence {
                                tunnel: [w266] -> w262
                                tunnel: [w265] -> w261
                                tunnel: [w264] -> w260
                                tunnel: w261 -> [w272]
                                tunnel: w260 -> [w271]
                                frame #0 {
                                w263 = 0 ("index")
                                # "this doesn't look\nmodular-allcards\nchannels and compare\nall parameters"
                                n261 = local read "OSC Configuration Control"() -> (w266:T6)
                                n262 = global read "Lock-in Globles Multiple Inputs and Outputs.vi" "OSC Configuration"() -> (w265:T9)
                                n263 = Subtract(x=w265, y=w266) -> (x-y=w270:T11)
                                n264 = Index Array(array=w270, index (row)=w263, index (col)=w263) -> (element=w269:T12)
                                n265 = Unbundle(w269) -> (w268:dbl)  [unwired: 4 out]
                                n266 = Equal?(x=w268, y=0.0) -> (x = y?=w264:bool)
                                }
                                frame #1 {
                                n267 = case shown="False" w271 {
                                tunnel: w272 -> [w274 w275]
                                frame False {
                                n268 = local write "OSC Configuration Control"(w274) -> ()
                                n269 = global write "Lock-in Globles Multiple Inputs and Outputs.vi" "Reset Lockin"(TRUE ("Reset Lockin")) -> ()
                                }
                                frame True {
                                n270 = local write "OSC Configuration Control"(w275) -> ()
                                }
                                }
                                }
                              }
                            }
                          }
                          n271 = global write "Lock-in Globles Multiple Inputs and Outputs.vi" "Input signal"(w225) -> ()
                          n272 = Get Date/Time In Seconds() -> (seconds since 1Jan1904=w237:timestamp)
                          n273 = global write "Lock-in Globles Multiple Inputs and Outputs.vi" "timestamp"(w237) -> ()
                          n274 = local read "AO Task"() -> (w230:refnum<k21>[])
                          n275 = local read "Sampling Information"() -> (w229:cluster{"Fs":dbl, "#s":dbl}[])
                          n276 = global read "Lock-in Globles Multiple Inputs and Outputs.vi" "Multiplication factor"() -> (w231:dbl)
                          n277 = call "Read and Return AO Task.vi"("OSC Configuration In"=w232, "AO Task In"=w230, "Sampling Information In"=w229, "Multiplication Factor In"=w231) -> ()  [unwired: 2 in]
                        }
                      }
                    }
                  }
                }
              }
            }
            frame 3 {
              # "will be true if it is taking a picture/producing\ndisplays and will be false if the program is\nwaiting"
              n278 = local read "Boolean_panel2"() -> (w276:bool)
              n279 = case shown="True" w276 {
                frame False {
                  # "no displays will be produced"
                }
                frame True {
                  n280 = local read "Remote"() -> (w328:bool)
                  n281 = case shown="True" w328 {
                    tunnel: [w339 w340] -> w327
                    frame False {
                      n282 = local read "OSC Configuration Control"() -> (w339:T6)
                    }
                    frame True {
                      n283 = global read "Lock-in Globles Multiple Inputs and Outputs.vi" "OSC Configuration"() -> (w340:T9)
                    }
                  }
                  n284 = local read "Phase&Tc Control"() -> (w305:T7)
                  n285 = local read "AI Block Size Control"() -> (w324:i32)
                  n286 = local read "Results"() -> (w323:dbl[][])
                  n287 = local read "Signal"() -> (w325:dbl[][])
                  n288 = local read "AI Rate"() -> (w326:dbl)
                  n289 = local read "Phase Log"() -> (w322:dbl[])
                  n290 = local read "Lockin Display D"() -> (w302:i16)
                  n291 = global read "Global Value_charles.vi" "Channel Setting 2"() -> (w318:T13)
                  n292 = call "Lock-In Analysis.vi"("Signal in"=w325, "Phase&Tc In"=w305, "AI Block Size In"=w324, "Results"=w323, "AI Rate In"=w326, "OSC Configuration In"=w327, "Phase Log In"=w322) -> ("Demodulation Out"=w319:dbl[][], "Phase Log Out"=w320:dbl[], "Phase&Tc Out"=w321:T1)  [unwired: 6 in]
                  n293 = local read "Display"() -> (w303:u16)
                  n294 = local write "Phase&Tc Control"(w321) -> ()
                  n295 = local read "Lockin Display A"() -> (w301:i16)
                  n296 = local write "Phase Log"(w320) -> ()
                  n297 = local read "Input Signals"() -> (w299:i16)
                  n298 = local read "Lockin Display B"() -> (w300:i16)
                  n299 = local read "Lockin Display C"() -> (w298:i16)
                  n300 = call "Produce Display.vi"("Channel Setting 2"=w318, "Demodulation In"=w319, "Display"=w303, "Input Signals In"=w299, "Lockin Display A In"=w301, "Lockin Display D In"=w302, "Lockin Display C In"=w298, "Lockin Display B In"=w300) -> ("Results"=w304:dbl[][], "Display Cluster (Not Into Cases) Out"=w306:T14, "Display Cluster (Into Cases) Out cluster"=w317:T15)  [unwired: 9 in]
                  n301 = Unbundle(w306) -> ("Array"=w295:dbl[], "Array 2"=w293:dbl[], "Array"=w294:dbl[], "Array 2"=w292:dbl[], "Array"=w290:dbl[], "Array 2"=w289:dbl[], "Array"=w291:dbl[], "Array 2"=w288:dbl[])  [unwired: 2 out]
                  n302 = local write "Display Y (or Theta) C"(w289) -> ()
                  n303 = local write "Display X (or R) C"(w290) -> ()
                  n304 = local read "Tab Control"() -> (w287:T2)
                  n305 = Unbundle(w317) -> ("Display 1"=w316:string, "Display 2"=w315:string, "Display 1"=w314:string, "Display 2"=w313:string, "Display 1"=w312:string, "Display 2"=w311:string, "Display 1"=w310:string, "Display 2"=w309:string, "Display 1"=w308:string, "Display 2"=w307:string)
                  n306 = local write "Display X (or R) A"(w295) -> ()
                  n307 = local write "Results"(w304) -> ()
                  n308 = global write "Lock-in Globles Multiple Inputs and Outputs.vi" "Results"(w304) -> ()
                  n309 = local write "Display Y (or Theta) D"(w288) -> ()
                  n310 = local write "Display X (or R) B"(w294) -> ()
                  n311 = case shown="\"Input Signals\"" w287 {
                    tunnel: w316 -> [w330 _ _ _ _]
                    tunnel: [w330 w332 w334 w336 w338] -> w297
                    tunnel: w315 -> [w329 _ _ _ _]
                    tunnel: [w329 w331 w333 w335 w337] -> w296
                    tunnel: w314 -> [_ w332 _ _ _]
                    tunnel: w313 -> [_ w331 _ _ _]
                    tunnel: w312 -> [_ _ w334 _ _]
                    tunnel: w311 -> [_ _ w333 _ _]
                    tunnel: w310 -> [_ _ _ w336 _]
                    tunnel: w309 -> [_ _ _ w335 _]
                    tunnel: w308 -> [_ _ _ _ w338]
                    tunnel: w307 -> [_ _ _ _ w337]
                    frame "Lock-in Display A", Default {
                    }
                    frame "Lock-in Display B" {
                    }
                    frame "Lock-in Display C" {
                    }
                    frame "Lock-in Display D" {
                    }
                    frame "Input Signals" {
                    }
                  }
                  n312 = local write "Display Y (or Theta) B"(w292) -> ()
                  n313 = local write "Display Y (or Theta) D"(w291) -> ()
                  n314 = local write "Display Y (or Theta) A"(w293) -> ()
                  n315 = local write "Display 1"(w297) -> ()
                  n316 = local write "Display 2"(w296) -> ()
                }
              }
              n317 = global read "Lock-in Globles Multiple Inputs and Outputs.vi" "Stop Lockin"() -> (w282:bool)
              n318 = local read "stop"() -> (w277:bool)
              n319 = global read "Lock-in Globles Multiple Inputs and Outputs.vi" "Reset Lockin"() -> (w286:bool)
              n320 = Or(x=w282, y=w277) -> (x .or. y?=w283:bool)
              n321 = Select(t=4.0 ("f"), s=w283, f=2.0) -> (s? t:f=w284:dbl)
              n322 = Select(t=5.0, s=w286, f=w284) -> (s? t:f=w278:dbl)
            }
            frame 4 {
              n323 = local read "AI Task"() -> (w343:refnum<k21>[])
              n324 = local read "AO Task"() -> (w342:refnum<k21>[])
              n325 = call "End Tasks.vi"("AO Task In"=w342, "AI Task In"=w343) -> ()  [unwired: 1 in]
              n326 = invoke on="stop" class="Bool (strict)" method="Reinit To Default"() -> ()  [unwired: 3 in, 3 out]
              n327 = property on="Read initial settings from:" class="Bool (strict)"("DisabledEnum"=T8."Enabled" ("Disabled")) -> ()  [unwired: 2 in, 2 out]
            }
            frame 5.. {
              n328 = local read "AI Task"() -> (w349:refnum<k21>[])
              n329 = local read "AO Task"() -> (w348:refnum<k21>[])
              n330 = call "End Tasks.vi"("AO Task In"=w348, "AI Task In"=w349) -> ()  [unwired: 1 in]
              n331 = invoke on="stop" class="Bool (strict)" method="Reinit To Default"() -> ()  [unwired: 3 in, 3 out]
            }
          }
        }
      }
      frame "Continuous", Default {
        w350 = T8."Enabled" ("Disabled")
        w351 = T8."Disabled and Grayed Out" ("Disabled")
        n332 = property on="Phase" class="DigNum (strict)"("DisabledEnum"=w350) -> ()  [unwired: 2 in, 2 out]
        n333 = property on="Frequency" class="DigNum (strict)"("DisabledEnum"=w350) -> ()  [unwired: 2 in, 2 out]
        n334 = property on="DC" class="DigNum (strict)"("DisabledEnum"=w350) -> ()  [unwired: 2 in, 2 out]
        n335 = property on="Signal Type" class="Enum (strict)"("DisabledEnum"=w350) -> ()  [unwired: 2 in, 2 out]
        n336 = property on="Amplitude" class="DigNum (strict)"("DisabledEnum"=w350) -> ()  [unwired: 2 in, 2 out]
        n337 = property on="Signal Type" class="Enum (strict)"("DisabledEnum"=w350) -> ()  [unwired: 2 in, 2 out]
        n338 = property on="Signal Button" class="Bool"("DisabledEnum"=w351) -> ()  [unwired: 2 in, 2 out]
        n339 = property on="Amp. button" class="Bool"("DisabledEnum"=w351) -> ()  [unwired: 2 in, 2 out]
        n340 = property on="DC Button" class="Bool"("DisabledEnum"=w351) -> ()  [unwired: 2 in, 2 out]
        n341 = property on="freq. button" class="Bool"("DisabledEnum"=w351) -> ()  [unwired: 2 in, 2 out]
        n342 = property on="Phase Button" class="Bool"("DisabledEnum"=w351) -> ()  [unwired: 2 in, 2 out]
        n343 = property on="Multiple Button" class="Bool"("DisabledEnum"=w351) -> ()  [unwired: 2 in, 2 out]
        n344 = while {
          shift-right: [w367] -> _
          shift-left: 0 -> [w359]
          tunnel: w357 -> [w365]
          tunnel: w356 -> [w364]
          tunnel: w355 -> [w363]
          tunnel: w354 -> [w362]
          tunnel: w353 -> [w361]
          tunnel: w352 -> [w360]
          stop <- w366 continue-if-true
          n345 = case shown="3" w359 {
            tunnel: [1 2 3 w493 w565 0.0 ("f")] -> w367
            tunnel: [TRUE TRUE TRUE TRUE FALSE TRUE] -> w366
            tunnel: w365 -> [w372 _ _ _ _ _]
            tunnel: w364 -> [w371 _ _ _ _ _]
            tunnel: w363 -> [_ w392 _ _ _ _]
            tunnel: w362 -> [_ w391 _ _ _ _]
            tunnel: w361 -> [_ w390 _ _ _ _]
            tunnel: w360 -> [_ w378 _ _ _ _]
            selector: w359 -> [_ _ _ _ w565 _]
            frame ..0, Default {
              w370 = FALSE ("Stop Lockin")
              # "sets up OSC configuration and AI configuration"
              n346 = local read "OSC Configuration Control"() -> (w375:T6)
              n347 = global write "Lock-in Globles Multiple Inputs and Outputs.vi" "Stop Lockin"(w370) -> ()
              n348 = global write "Lock-in Globles Multiple Inputs and Outputs.vi" "Reset Lockin"(w370) -> ()
              n349 = call "Configure Frequencies.vi"("OSC Configuration In"=w375) -> ("Frequency Out"=w373:dbl, "OSC Configuation Out"=w374:T9)  [unwired: 1 in]
              n350 = call "AI Configurations.vi"("Auto control  max AI rate/ AI block size"=w372, "Max AI Rate In"=w371, "Frequency In"=w373) -> ("AI Rate Out"=w368:i32, "AI Block Size Out"=w369:dbl)
              n351 = local write "OSC Configuration Control"(w374) -> ()
              n352 = global write "Lock-in Globles Multiple Inputs and Outputs.vi" "OSC Configuration"(w374) -> ()
              n353 = local write "AI Rate"(w368) -> ()
              n354 = local write "AI Block Size Control"(w369) -> ()
            }
            frame 1 {
              # "makes AI/AO task channels"
              # "gets the number of cards to\ncreate the necessary channels"
              n355 = local read "OSC Configuration Control"() -> (w382:T6)
              n356 = Array Size(array=w382) -> (size(s)=w381:i32[])
              n357 = Index Array(array=w381, index=0) -> (element=w379:i32)
              n358 = call "Make In, Out Channels.vi"("AI Configuration In"=w392, "AI Buffer Size (s) In"=w390, "AO Configuration Out"=w391, "Num. of Cards"=w379, "OSC Configuration In"=w382, "AI Block Size In"=w378) -> ("AI Task Out"=→"AI Task":refnum<k21>[], "AO Task Out"=→"AO Task":refnum<k21>[], "Phase Log Out"=→"Phase Log":dbl[], "AI Rate Out"=→"AI Rate":dbl, "Sampling Information Out"=w386:cluster{"Fs":dbl, "#s":dbl}[])  [unwired: 5 in]
              "Sampling Information" <- w386
              n359 = global write "Lock-in Globles Multiple Inputs and Outputs.vi" "Sampling information"(w386) -> ()
            }
            frame 2 {
              # "makes sure phase array is read w/ USB-4431"
              # "produces input signal/graph"
              # "event for the buttons, doesn't impact functionality"
              # "all of these are settings for the buttons"
              n360 = local read "Numeric_Card"() -> (w399:dbl)
              n361 = property on="Numeric_Channel" class="DigNum (strict)"("Visible"=FALSE) -> ()  [unwired: 2 in, 2 out]
              n362 = local read "Numeric_Channel"() -> (w398:dbl)
              n363 = property on="Numeric_Card" class="DigNum (strict)"("Visible"=FALSE) -> ()  [unwired: 2 in, 2 out]
              n364 = event shown="[0] Timeout" {
                selector: _ -> [_ _ _ _ _]
                dyn-events: _ -> [_ _ _ _ _]
                timeout: 1 -> [_ _ _ _ _]
                tunnel: w399 -> [_ w424 w430 w433 w438]
                tunnel: w398 -> [_ _ _ w436 w440]
                tunnel: "OSC Configuration Control" -> [w420 w421 w426 w431 w437]
                tunnel: [w420 w421 w426 w431 w437] -> w394
                event Timeout {
                  n365 = event-data() -> ()  [unwired: 1 in, 2 out]
                }
                event "Next_Card": Value Change {
                  n366 = event-data() -> ()  [unwired: 1 in, 2 out]
                  n367 = Add(x=1.0, y=w424) -> (x+y=w423:dbl)
                  n368 = local write "Numeric_Card"(w423) -> ()
                  n369 = Build Array(w423) -> (w422:dbl[])
                  n370 = property on="OSC Configuration Control" class="Arr (strict)"("Index Values"=w422) -> ()  [unwired: 2 in, 2 out]
                }
                event "Previous_Card": Value Change {
                  n371 = event-data() -> ()  [unwired: 1 in, 2 out]
                  n372 = Subtract(x=w430, y=1.0) -> (x-y=w428:dbl)
                  n373 = local write "Numeric_Card"(w428) -> ()
                  n374 = Build Array(w428) -> (w427:dbl[])
                  n375 = property on="OSC Configuration Control" class="Arr (strict)"("Index Values"=w427) -> ()  [unwired: 2 in, 2 out]
                }
                event "Next_Channel": Value Change {
                  n376 = event-data() -> ()  [unwired: 1 in, 1 out]
                  n377 = Add(x=1.0, y=w436) -> (x+y=w434:dbl)
                  n378 = local write "Numeric_Channel"(w434) -> ()
                  n379 = Build Array(w433, w434) -> (w432:dbl[])
                  n380 = property on="OSC Configuration Control" class="Arr (strict)"("Index Values"=w432) -> ()  [unwired: 2 in, 2 out]
                }
                event "Previous_Channel": Value Change {
                  n381 = event-data() -> ()  [unwired: 1 in, 1 out]
                  n382 = Subtract(x=w440, y=1.0) -> (x-y=w441:dbl)
                  n383 = local write "Numeric_Channel"(w441) -> ()
                  n384 = Build Array(w438, w441) -> (w442:dbl[])
                  n385 = property on="OSC Configuration Control" class="Arr (strict)"("Index Values"=w442) -> ()  [unwired: 2 in, 2 out]
                }
              }
              n386 = local read "loop counter"() -> (w393:dbl)
              n387 = case shown="1" w393 {
                frame 0, Default {
                  n388 = local read "loop counter"() -> (w415:dbl)
                  n389 = Increment(x=w415) -> (x+1=w416:dbl)
                  n390 = local write "loop counter"(w416) -> ()
                }
                frame 1 {
                  n391 = local read "loop counter"() -> (w417:dbl)
                  n392 = local read "Phase&Tc Control 2"() -> (w419:T1)
                  n393 = local write "Phase&Tc Control"(w419) -> ()
                  n394 = Increment(x=w417) -> (x+1=w418:dbl)
                  n395 = local write "loop counter"(w418) -> ()
                }
              }
              n396 = local read "AI Buffer Size (s) Control"() -> (w409:i32)
              n397 = local read "AI Block Size Control"() -> (w410:i32)
              n398 = local read "AI Rate"() -> (w408:dbl)
              n399 = local read "AI Task"() -> (w411:refnum<k21>[])
              n400 = call "Read and Return AI Task.vi"("AI Task In"=w411, "AI Block Size In"=w410, "AI Buffer Size (s) In"=w409, "AI Rate In"=w408) -> ("Input Signal Out"=w407:dbl[][], "Backlog Out"=→"Backlog":u8)  [unwired: 2 in]
              "Input Signal" <- w407
              "Signal" <- w407
              n401 = global write "Lock-in Globles Multiple Inputs and Outputs.vi" "Input signal"(w407) -> ()
              n402 = case shown="False" "Remote" {
                tunnel: [w444 w467] -> w404
                tunnel: w394 -> [w443 _]
                frame False {
                  n403 = Index Array(array=w443, index (row)=0, index (col)=0 ("disabled index (col)")) -> (element=w448:T10)
                  n404 = Unbundle By Name(w448) -> ("Frequency"=w447:dbl)
                  n405 = for {
                    tunnel: w447 -> [w453]
                    tunnel: w443 -> [w452] mode=indexing
                    tunnel: [w451] -> w444 mode=indexing
                    i -> [w450]
                    n406 = Equal To 0?(x=w450) -> (x = 0?=w449:bool)
                    n407 = for {
                      tunnel: w452 -> [w460] mode=indexing
                      tunnel: w453 -> [w459]
                      tunnel: [w458] -> w451 mode=indexing
                      tunnel: w449 -> [w454]
                      i -> [w456]
                      n408 = Equal To 0?(x=w456) -> (x = 0?=w455:bool)
                      n409 = And(x=w455, y=w454) -> (x .and. y?=w457:bool)
                      n410 = case shown="True" w457 {
                        tunnel: w460 -> [w463 w464]
                        tunnel: w459 -> [w462 _]
                        tunnel: [w461 w464] -> w458
                        frame False {
                          n411 = Bundle By Name(cluster=w463, "Frequency"=w462) -> (w461:T10)
                        }
                        frame True {
                        }
                      }
                    }
                  }
                  n412 = local write "OSC Configuration Control"(w444) -> ()
                  n413 = global write "Lock-in Globles Multiple Inputs and Outputs.vi" "OSC Configuration"(w444) -> ()
                }
                frame True {
                  n414 = flat-sequence {
                    tunnel: [w471] -> w467
                    tunnel: [w470] -> w466
                    tunnel: [w469] -> w465
                    tunnel: w466 -> [w477]
                    tunnel: w465 -> [w476]
                    frame #0 {
                      w468 = 0 ("index")
                      n415 = local read "OSC Configuration Control"() -> (w471:T6)
                      n416 = global read "Lock-in Globles Multiple Inputs and Outputs.vi" "OSC Configuration"() -> (w470:T9)
                      n417 = Subtract(x=w470, y=w471) -> (x-y=w475:T11)
                      n418 = Index Array(array=w475, index (row)=w468, index (col)=w468) -> (element=w474:T12)
                      n419 = Unbundle(w474) -> (w473:dbl)  [unwired: 4 out]
                      n420 = Equal?(x=w473, y=0.0) -> (x = y?=w469:bool)
                    }
                    frame #1 {
                      n421 = case shown="False" w476 {
                        tunnel: w477 -> [w479 w480]
                        frame False {
                          n422 = local write "OSC Configuration Control"(w479) -> ()
                          n423 = global write "Lock-in Globles Multiple Inputs and Outputs.vi" "Reset Lockin"(TRUE ("Reset Lockin")) -> ()
                        }
                        frame True {
                          n424 = local write "OSC Configuration Control"(w480) -> ()
                        }
                      }
                    }
                  }
                }
              }
              n425 = Get Date/Time In Seconds() -> (seconds since 1Jan1904=w414:timestamp)
              n426 = global write "Lock-in Globles Multiple Inputs and Outputs.vi" "timestamp"(w414) -> ()
              n427 = local read "AO Task"() -> (w402:refnum<k21>[])
              n428 = local read "Sampling Information"() -> (w401:cluster{"Fs":dbl, "#s":dbl}[])
              n429 = global read "Lock-in Globles Multiple Inputs and Outputs.vi" "Multiplication factor"() -> (w403:dbl)
              n430 = call "Read and Return AO Task.vi"("OSC Configuration In"=w404, "AO Task In"=w402, "Sampling Information In"=w401, "Multiplication Factor In"=w403) -> ()  [unwired: 2 in]
            }
            frame 3 {
              # "makes sure phase array\nis read in USB-4431"
              # "event for buttons"
              # "button config."
              n431 = property on="Numeric_OSC" class="DigNum (strict)"("Visible"=FALSE) -> ()  [unwired: 2 in, 2 out]
              n432 = local read "Remote"() -> (w537:bool)
              n433 = local read "Numeric_OSC"() -> (w484:dbl)
              n434 = case shown="True" w537 {
                tunnel: [w560 w561] -> w536
                frame False {
                  n435 = local read "OSC Configuration Control"() -> (w560:T6)
                }
                frame True {
                  n436 = global read "Lock-in Globles Multiple Inputs and Outputs.vi" "OSC Configuration"() -> (w561:T9)
                }
              }
              n437 = event shown="[0] Timeout" {
                selector: _ -> [_ _ _]
                dyn-events: _ -> [_ _ _]
                timeout: 1 -> [_ _ _]
                tunnel: w484 -> [_ _ _]
                tunnel: "Phase&Tc Control" -> [w539 w540 w545]
                tunnel: [w539 w540 w545] -> w483
                event Timeout {
                  n438 = event-data() -> ()  [unwired: 1 in, 2 out]
                }
                event "Next_OSC": Value Change {
                  n439 = event-data() -> ()  [unwired: 1 in, 1 out]
                  n440 = local read "Numeric_OSC"() -> (w543:dbl)
                  n441 = Add(x=1.0, y=w543) -> (x+y=w542:dbl)
                  n442 = local write "Numeric_OSC"(w542) -> ()
                  n443 = Build Array(w542) -> (w541:dbl[])
                  n444 = property on="Phase&Tc Control" class="Arr (strict)"("Index Values"=w541) -> ()  [unwired: 2 in, 2 out]
                }
                event "Previous_OSC": Value Change {
                  n445 = event-data() -> ()  [unwired: 1 in, 1 out]
                  n446 = local read "Numeric_OSC"() -> (w547:dbl)
                  n447 = Subtract(x=w547, y=1.0) -> (x-y=w549:dbl)
                  n448 = local write "Numeric_OSC"(w549) -> ()
                  n449 = Build Array(w549) -> (w548:dbl[])
                  n450 = property on="Phase&Tc Control" class="Arr (strict)"("Index Values"=w548) -> ()  [unwired: 2 in, 2 out]
                }
              }
              n451 = local read "AI Block Size Control"() -> (w533:i32)
              n452 = local read "Results"() -> (w532:dbl[][])
              n453 = local read "Signal"() -> (w534:dbl[][])
              n454 = local read "AI Rate"() -> (w535:dbl)
              n455 = local read "Phase Log"() -> (w531:dbl[])
              n456 = local read "loop counter"() -> (w481:dbl)
              n457 = global read "Global Value_charles.vi" "Channel Setting 2"() -> (w527:T13)
              n458 = call "Lock-In Analysis.vi"("Signal in"=w534, "Phase&Tc In"=w483, "AI Block Size In"=w533, "Results"=w532, "AI Rate In"=w535, "OSC Configuration In"=w536, "Phase Log In"=w531) -> ("Demodulation Out"=w528:dbl[][], "Phase Log Out"=w529:dbl[], "Phase&Tc Out"=w530:T1)  [unwired: 6 in]
              n459 = case shown="1, Default" w481 {
                tunnel: "Phase&Tc Control" -> [w538 _]
                frame 0 {
                  "Phase&Tc Control 2" <- w538
                }
                frame 1, Default {
                }
              }
              n460 = local write "Phase&Tc Control"(w530) -> ()
              n461 = local write "Phase Log"(w529) -> ()
              n462 = global read "Lock-in Globles Multiple Inputs and Outputs.vi" "Stop Lockin"() -> (w497:bool)
              n463 = call "Produce Display.vi"("Channel Setting 2"=w527, "Demodulation In"=w528, "Display"="Display", "Input Signals In"="Input Signals", "Lockin Display A In"="Lockin Display A", "Lockin Display D In"="Lockin Display D", "Lockin Display C In"="Lockin Display C", "Lockin Display B In"="Lockin Display B") -> ("Results"=w526:dbl[][], "Display Cluster (Not Into Cases) Out"=w512:T14, "Display Cluster (Into Cases) Out cluster"=w523:T15)  [unwired: 9 in]
              "Results" <- w526
              n464 = global read "Lock-in Globles Multiple Inputs and Outputs.vi" "Reset Lockin"() -> (w502:bool)
              n465 = Or(x=w497, y="stop") -> (x .or. y?=w499:bool)
              n466 = Unbundle(w512) -> ("Array"=→"Display X (or R) A":dbl[], "Array 2"=→"Display Y (or Theta) A":dbl[], "Array"=→"Display X (or R) B":dbl[], "Array 2"=→"Display Y (or Theta) B":dbl[], "Array"=→"Display X (or R) C":dbl[], "Array 2"=→"Display Y (or Theta) C":dbl[], "Array"=→"Display X (or R) D":dbl[], "Array 2"=→"Display Y (or Theta) D":dbl[])  [unwired: 2 out]
              n467 = Unbundle(w523) -> ("Display 1"=w522:string, "Display 2"=w521:string, "Display 1"=w520:string, "Display 2"=w519:string, "Display 1"=w518:string, "Display 2"=w517:string, "Display 1"=w516:string, "Display 2"=w515:string, "Display 1"=w514:string, "Display 2"=w513:string)
              n468 = global write "Lock-in Globles Multiple Inputs and Outputs.vi" "Results"(w526) -> ()
              n469 = Select(t=4.0 ("f"), s=w499, f=2.0) -> (s? t:f=w500:dbl)
              n470 = case shown="\"Input Signals\"" "Tab Control" {
                tunnel: w522 -> [w551 _ _ _ _]
                tunnel: [w551 w553 w555 w557 w559] -> w525
                tunnel: w521 -> [w550 _ _ _ _]
                tunnel: [w550 w552 w554 w556 w558] -> w524
                tunnel: w520 -> [_ w553 _ _ _]
                tunnel: w519 -> [_ w552 _ _ _]
                tunnel: w518 -> [_ _ w555 _ _]
                tunnel: w517 -> [_ _ w554 _ _]
                tunnel: w516 -> [_ _ _ w557 _]
                tunnel: w515 -> [_ _ _ w556 _]
                tunnel: w514 -> [_ _ _ _ w559]
                tunnel: w513 -> [_ _ _ _ w558]
                frame "Lock-in Display A", Default {
                }
                frame "Lock-in Display B" {
                }
                frame "Lock-in Display C" {
                }
                frame "Lock-in Display D" {
                }
                frame "Input Signals" {
                }
              }
              "Display 2" <- w524
              "Display 1" <- w525
              n471 = Select(t=5.0, s=w502, f=w500) -> (s? t:f=w493:dbl)
            }
            frame 4 {
              # "resets the stop button"
              n472 = local read "AI Task"() -> (w563:refnum<k21>[])
              n473 = local read "AO Task"() -> (w562:refnum<k21>[])
              n474 = call "End Tasks.vi"("AO Task In"=w562, "AI Task In"=w563) -> ()  [unwired: 1 in]
              n475 = invoke on="stop" class="Bool (strict)" method="Reinit To Default"() -> ()  [unwired: 3 in, 3 out]
            }
            frame 5.. {
              # "resets the stop button"
              n476 = local read "AI Task"() -> (w569:refnum<k21>[])
              n477 = local read "AO Task"() -> (w568:refnum<k21>[])
              n478 = call "End Tasks.vi"("AO Task In"=w568, "AI Task In"=w569) -> ()  [unwired: 1 in]
              n479 = invoke on="stop" class="Bool (strict)" method="Reinit To Default"() -> ()  [unwired: 3 in, 3 out]
            }
          }
        }
      }
    }
  }
  "loop counter" <- 0.0 ("loop counter")
